vi "XY_plot_BW_gnuplot_DFT.vi"(0 "Plot Array":cluster{dbl[], dbl[]}[](array[cluster])=[{[-60.0, -57.5, -55.0, -52.5, -50.0, -47.5, -45.0, -42.5, -40.0, -37.5, -35.0, -32.5, -30.0, -27.5, -25.0, -22.5, -20.0, -17.5, -15.0, -12.5, -10.0, -7.5, -5.0, -2.5, 0.0, 2.5, 5.0, 7.5, 10.0, 12.5, 15.0, 17.5, 20.0, 22.5, 25.0, 27.5, 30.0, 32.5, 35.0, 37.5, 40.0, 42.5, 45.0, 47.5, 50.0, 52.5, 55.0, 57.5, 60.0], [0.6926572, 0.7210577, 0.7336973, 0.7296005, 0.7065726, 0.6675372, 0.6509055, 0.666809, 0.7019418, 0.7280011, 0.7366155, 0.7266001, 0.6985851, 0.6651901, 0.6448196, 0.6503613, 0.6875361, 0.7183487, 0.7265879, 0.7127957, 0.6835807, 0.6433804, 0.621768, 0.6334316, 0.670315, 0.7004812, 0.7073965, 0.6966882, 0.6633028, 0.6324072, 0.6188318, 0.6325043, 0.6686596, 0.7028522, 0.7124769, 0.7009745, 0.6723148, 0.6300974, 0.6088247, 0.6211135, 0.6589306, 0.6947777, 0.7073037, 0.6986245, 0.6763866, 0.6414574, 0.6211717, 0.6351113, 0.6695351]}, {[-250.0, -245.0, -240.0, -235.0, -230.0, -225.0, -220.0, -215.0, -210.0, -205.0, -200.0, -195.0, -190.0, -185.0, -180.0, -175.0, -170.0, -165.0, -160.0, -155.0, -150.0, -145.0, -140.0, -135.0, -130.0, -125.0, -120.0, -115.0, -110.0, -105.0, -100.0, -95.0, -90.0, -85.0, -80.0, -75.0, -70.0, -65.0, -60.0, -55.0, -50.01, -45.0, -40.0, -35.0, -30.0, -25.0, -20.0, -15.0, -10.0, -5.0, 0.0, 5.0, 10.0, 15.0, 20.0, 25.0, 30.0, 35.0, 40.0, 45.0, 50.0, 55.0, 60.0, 65.0, 70.0, 75.0, 80.0, 85.0, 90.0, 95.0, 100.0, 105.0, 110.0, 115.0, 120.0, 125.0, 130.0, 135.0, 140.0, 145.0, 150.0, 155.0, 160.0, 165.0, 170.0, 175.0, 180.0, 185.0, 190.0, 195.0, 200.0, 205.0, 210.0, 215.0, 220.0, 225.0, 230.0, 235.0, 240.0, 245.0, 250.0], [0.6258228, 0.6506318, 0.6351729, 0.7010563, 0.666653, 0.6318866, 0.6418648, 0.6775528, 0.6772554, 0.6566841, 0.6714944, 0.6985058, 0.678455, 0.6443694, 0.6531426, 0.6719725, 0.6524493, 0.6260805, 0.64483, 0.6829994, 0.659875, 0.6199248, 0.6366962, 0.6786398, 0.6778554, 0.6498207, 0.6635327, 0.6868778, 0.6697222, 0.641235, 0.6519968, 0.6776285, 0.6615762, 0.6471135, 0.6708456, 0.6800422, 0.6428301, 0.6228845, 0.6529464, 0.6825998, 0.6581101, 0.6411269, 0.673482, 0.6917087, 0.6575879, 0.6369717, 0.6618911, 0.6765118, 0.6419686, 0.6179553, 0.6401561, 0.6835365, 0.6558098, 0.6374033, 0.6669807, 0.6870508, 0.6587676, 0.6427578, 0.6715876, 0.6928693, 0.6606558, 0.6407446, 0.6661822, 0.6808485, 0.649376, 0.6387559, 0.6726195, 0.6840063, 0.6428675, 0.6274834, 0.6671746, 0.6892811, 0.6632424, 0.6494314, 0.6844879, 0.7061464, 0.667844, 0.6523467, 0.6754834, 0.6831993, 0.6537409, 0.650146, 0.6863526, 0.6915197, 0.6527784, 0.6421613, 0.6812965, 0.7003779, 0.6678409, 0.6625075, 0.6991244, 0.6979552, 0.658929, 0.6426513, 0.6723225, 0.6756767, 0.6454689, 0.6509592, 0.6810775, 0.6720489, 0.6356013]}, {[-250.0, -245.0, -240.0, -235.0, -230.0, -225.0, -220.0, -215.0, -210.0, -205.0, -200.0, -195.0, -190.0, -185.0, -180.0, -175.0, -170.0, -165.0, -160.0, -155.0, -150.0, -145.0, -140.0, -135.0, -130.0, -125.0, -120.0, -115.0, -110.0, -105.0, -100.0, -95.0, -90.0, -85.0, -80.0, -75.0, -70.0, -65.0, -60.0, -55.0, -50.0, -45.0, -40.0, -35.0, -30.0, -25.0, -20.0, -15.0, -10.0, -5.0, 0.0, 5.0, 10.0, 15.0, 20.0, 25.0, 30.0, 35.0, 40.0, 45.0, 50.0, 55.0, 60.0, 65.0, 70.0, 75.0, 80.0, 85.0, 90.0, 95.0, 100.0, 105.0, 110.0, 115.0, 120.0, 125.0, 130.0, 135.0, 140.0, 145.0, 150.0, 155.0, 160.0, 165.0, 170.0, 175.0, 180.0, 185.0, 190.0, 195.0, 200.0, 205.0, 210.0, 215.0, 220.0, 225.0, 230.0, 235.0, 240.0, 245.0, 250.0], [0.7199633, 0.71586, 0.7146621, 0.720776, 0.7208473, 0.7155022, 0.7097559, 0.7138091, 0.7261716, 0.7358918, 0.7412903, 0.7471439, 0.7430872, 0.7318501, 0.7242517, 0.7215749, 0.7168437, 0.7096065, 0.7113085, 0.7181352, 0.7186632, 0.7101602, 0.7056491, 0.713961, 0.727691, 0.7317399, 0.7345805, 0.7315234, 0.7289434, 0.7173446, 0.7110098, 0.7114931, 0.7136913, 0.7211985, 0.72029, 0.7193148, 0.7070549, 0.6992863, 0.7012733, 0.7126021, 0.7232668, 0.7273864, 0.7349982, 0.7363434, 0.7267652, 0.7217994, 0.7205206, 0.7193069, 0.7106847, 0.6995876, 0.6970152, 0.7001581, 0.6993276, 0.6998134, 0.7069099, 0.7110891, 0.7119888, 0.7107461, 0.7153481, 0.7219045, 0.714913, 0.7080906, 0.7068127, 0.7038392, 0.698503, 0.7005704, 0.7003845, 0.7038539, 0.6953904, 0.6920397, 0.7001599, 0.7094703, 0.7137769, 0.7180073, 0.7230059, 0.7250995, 0.7213451, 0.7111041, 0.7094518, 0.7083167, 0.7040226, 0.7066045, 0.7097009, 0.7077949, 0.7014225, 0.7058737, 0.7102084, 0.7183272, 0.7217187, 0.7251733, 0.7275464, 0.7183908, 0.7059657, 0.7016548, 0.7006334, 0.702877, 0.7023345, 0.7034203, 0.7042745, 0.698976, 0.6924951]}, {[-250.0, -245.0, -240.0, -235.0, -230.0, -225.0, -220.0, -215.0, -210.0, -205.0, -200.0, -195.0, -190.0, -185.0, -180.0, -175.0, -170.0, -165.0, -160.0, -155.0, -150.0, -145.0, -140.0, -135.0, -130.0, -125.0, -120.0, -115.0, -110.0, -105.0, -100.0, -95.0, -90.0, -85.0, -80.0, -75.0, -70.0, -65.0, -60.0, -55.0, -50.0, -45.0, -40.0, -35.0, -30.0, -25.0, -20.0, -15.0, -10.0, -5.0, 0.0, 5.0, 10.0, 15.0, 20.0, 25.0, 30.0, 35.0, 40.0, 45.0, 50.0, 55.0, 60.0, 65.0, 70.0, 75.0, 80.0, 85.0, 90.0, 95.0, 100.0, 105.0, 110.0, 115.0, 120.0, 125.0, 130.0, 135.0, 140.0, 145.0, 150.0, 155.0, 160.0, 165.0, 170.0, 175.0, 180.0, 185.0, 190.0, 195.0, 200.0, 205.0, 210.0, 215.0, 220.0, 225.0, 230.0, 235.0, 240.0, 245.0, 250.0], [0.768425, 0.7646976, 0.7648598, 0.7620641, 0.7619677, 0.7591337, 0.7573157, 0.7577341, 0.7682732, 0.7776914, 0.7864129, 0.7911217, 0.7902806, 0.7870794, 0.7748631, 0.7664278, 0.7640868, 0.7634201, 0.7630689, 0.7622264, 0.7616281, 0.763408, 0.764395, 0.7665321, 0.771622, 0.7807466, 0.7826597, 0.784532, 0.7764856, 0.7691938, 0.7589803, 0.7538694, 0.7541752, 0.7570843, 0.7569958, 0.753328, 0.7533831, 0.7480442, 0.7493855, 0.7557662, 0.768794, 0.7812232, 0.7894507, 0.7928332, 0.7911097, 0.7813342, 0.7759887, 0.7691784, 0.7640505, 0.7602281, 0.7583228, 0.753628, 0.7548767, 0.7528715, 0.7584033, 0.7654095, 0.7705307, 0.7787003, 0.7801007, 0.7821146, 0.7765937, 0.768884, 0.7656759, 0.7562703, 0.7536232, 0.7539161, 0.7465613, 0.7489434, 0.7465653, 0.7487705, 0.7513418, 0.7602761, 0.771601, 0.779764, 0.7822907, 0.78155, 0.7763815, 0.7693112, 0.7626131, 0.7605712, 0.7588274, 0.7591805, 0.7584174, 0.7597108, 0.7548346, 0.7577244, 0.7606031, 0.7694007, 0.7775843, 0.7796888, 0.7780972, 0.7765036, 0.7638986, 0.760308, 0.7578089, 0.7541802, 0.7539944, 0.7565544, 0.7576207, 0.7557231, 0.7539951]}, {[-250.0, -240.0, -230.0, -220.0, -210.0, -200.0, -190.0, -180.0, -170.0, -160.0, -150.0, -140.0, -130.0, -120.0, -110.0, -100.0, -90.0, -80.0, -70.0, -60.0, -50.0, -40.0, -30.0, -20.0, -10.0, 0.0, 10.0, 20.0, 30.0, 40.0, 50.0, 60.0, 70.0, 80.0, 90.0, 100.0, 110.0, 120.0, 130.0, 140.0, 150.0, 160.0, 170.0, 180.0, 190.0, 200.0, 210.0, 220.0, 230.0, 240.0, 250.0], [0.7802652, 0.7730503, 0.7695233, 0.768015, 0.7807572, 0.7935942, 0.7974301, 0.7898797, 0.7780562, 0.7727421, 0.7754456, 0.7827163, 0.792625, 0.796434, 0.7864364, 0.7709765, 0.7651486, 0.7583434, 0.7591986, 0.7686091, 0.7853258, 0.8037569, 0.8016167, 0.7895253, 0.7775238, 0.7695855, 0.7682042, 0.7766473, 0.7899663, 0.7972402, 0.7915579, 0.78097, 0.7681623, 0.7627507, 0.7612609, 0.7754872, 0.7942263, 0.8006955, 0.7949862, 0.7807588, 0.7743586, 0.7702566, 0.7745907, 0.7822656, 0.7926563, 0.7935593, 0.7845497, 0.7732503, 0.7678837, 0.7717659, 0.773242]}, {[-250.0, -240.0, -230.0, -220.0, -210.0, -200.0, -190.0, -180.0, -170.0, -160.0, -150.0, -140.0, -130.0, -120.0, -110.0, -100.0, -90.0, -80.0, -70.0, -60.0, -50.0, -40.0, -30.0, -20.0, -10.0, 0.0, 10.0, 20.0, 30.0, 40.0, 50.0, 60.0, 70.0, 80.0, 90.0, 100.0, 110.0, 120.0, 130.0, 140.0, 150.0, 160.0, 170.0, 180.0, 190.0, 200.0, 210.0, 220.0, 230.0, 240.0, 250.0], [0.7879372, 0.7788166, 0.7776735, 0.7776241, 0.7889971, 0.8028856, 0.8070604, 0.8038303, 0.7927997, 0.7844949, 0.7865187, 0.7911869, 0.8018413, 0.8059924, 0.7943886, 0.7807321, 0.7705954, 0.7683053, 0.7699354, 0.779466, 0.7983266, 0.8136788, 0.8131328, 0.8038514, 0.7875963, 0.7800124, 0.7816548, 0.7885765, 0.8014482, 0.8085178, 0.8013688, 0.7883396, 0.7755844, 0.7736845, 0.7744691, 0.7907869, 0.8086567, 0.8114194, 0.8067535, 0.7936511, 0.7873925, 0.7810313, 0.7904059, 0.7965633, 0.8057665, 0.8044745, 0.7962059, 0.788702, 0.7812019, 0.7861557, 0.7902221]}, {[-250.0, -240.0, -230.0, -220.0, -210.0, -200.0, -190.0, -180.0, -170.0, -160.0, -150.0, -140.0, -130.0, -120.0, -110.0, -100.0, -90.0, -80.0, -70.0, -60.0, -50.0, -40.0, -30.0, -20.0, -10.0, 0.0, 10.0, 20.0, 30.0, 40.0, 50.0, 60.0, 70.0, 80.0, 90.0, 100.0, 110.0, 120.0, 130.0, 140.0, 150.0, 160.0, 170.0, 180.0, 190.0, 200.0, 210.0, 220.0, 230.0, 240.0, 250.0], [0.8154395, 0.8122923, 0.8086691, 0.8108997, 0.8191707, 0.8265118, 0.8294095, 0.8293452, 0.822631, 0.8238484, 0.8233996, 0.8241853, 0.8276184, 0.8234715, 0.8165378, 0.8082245, 0.798939, 0.798317, 0.8042167, 0.8193354, 0.8322321, 0.8402989, 0.8372588, 0.8290143, 0.8194996, 0.8153282, 0.8137867, 0.821221, 0.8254559, 0.8235515, 0.8236829, 0.8128044, 0.8098797, 0.8100971, 0.8177005, 0.8258541, 0.8346069, 0.8371071, 0.8288949, 0.8221575, 0.8182937, 0.8175638, 0.8224113, 0.8234351, 0.8289554, 0.824578, 0.819657, 0.8128183, 0.8152596, 0.8195102, 0.8255393]}, {[-250.0, -240.0, -230.0, -220.0, -210.0, -200.0, -190.0, -180.0, -170.0, -160.0, -150.0, -140.0, -130.0, -120.0, -110.0, -100.0, -90.0, -80.0, -70.0, -60.0, -50.0, -40.0, -30.0, -20.0, -10.0, 0.0, 10.0, 20.0, 30.0, 40.0, 50.0, 60.0, 70.0, 80.0, 90.0, 100.0, 110.0, 120.0, 130.0, 140.0, 150.0, 160.0, 170.0, 180.0, 190.0, 200.0, 210.0, 220.0, 230.0, 240.0, 250.0], [0.83059, 0.8293368, 0.8266022, 0.8290301, 0.8318731, 0.8391975, 0.8396511, 0.8408702, 0.8420259, 0.8377043, 0.837982, 0.8357183, 0.8335366, 0.8289886, 0.8236064, 0.8201522, 0.8188415, 0.8206514, 0.8238208, 0.8296316, 0.8366576, 0.8424445, 0.8437929, 0.8414023, 0.8376481, 0.8330458, 0.8310008, 0.8321893, 0.8334765, 0.832358, 0.8307255, 0.8322423, 0.8301097, 0.8318011, 0.8373023, 0.8428455, 0.8447038, 0.843124, 0.8437177, 0.8434732, 0.8408547, 0.8400876, 0.8407896, 0.8403817, 0.8420662, 0.8382707, 0.8379485, 0.8372055, 0.8393238, 0.8426629, 0.8465353]}] {"?" format="%.2f"; "?" format="%.2f"}, 1 "Job Directory":path=path "/G5_1_HD/Users/paulhayden/Desktop/Ryan/8-5-06") -> (2 "Saved Automatically?":bool, 3 "Tex Info String":string="set term epslatex\nset output \"Plot.eps\"\nset xlabel '$Wavelength~[mm]$'\nset ylabel '$U/Ur~Spectral~energy$'\nset samples 1000\nset pointsize 1.00\nset title '$$' 0, 0\nset size 0.75,2.5\n\n#set key 225, -696.080\n unset key\n set xrange [0 : 250] \n# set autoscale x \n set yrange [-602 : 84]\n# set autoscale y \nset ytics (\"x/h=313\" 0,\"x/h=218\" -84,\"x/h=124\" -168,\"x/h=102\" -252,\"x/h=66\" -336,\"x/h=34\" -420,\"x/h=18\" -504,\"x/h=10\" -588)\n\nplot \"Spec_U_Ur_x_h_10_x_h_18d.dat\" index 0 using 1:2 axes x1y1 title '$x/h=313$' with linespoints, \\\n\"Spec_U_Ur_x_h_10_x_h_18d.dat\" index 1 using 1:2 axes x1y1 title '$x/h=218$' with linespoints, \\\n\"Spec_U_Ur_x_h_10_x_h_18d.dat\" index 2 using 1:2 axes x1y1 title '$x/h=124$' with linespoints, \\\n\"Spec_U_Ur_x_h_10_x_h_18d.dat\" index 3 using 1:2 axes x1y1 title '$x/h=102$' with linespoints, \\\n\"Spec_U_Ur_x_h_10_x_h_18d.dat\" index 4 using 1:2 axes x1y1 title '$x/h=66$' with linespoints, \\\n\"Spec_U_Ur_x_h_10_x_h_18d.dat\" index 5 using 1:2 axes x1y1 title '$x/h=34$' with linespoints, \\\n\"Spec_U_Ur_x_h_10_x_h_18d.dat\" index 6 using 1:2 axes x1y1 title '$x/h=18$' with linespoints, \\\n\"Spec_U_Ur_x_h_10_x_h_18d.dat\" index 7 using 1:2 axes x1y1 title '$x/h=10$' with linespoints", 4 "Plot data file":path)   [LabVIEW 2010]
uses:
  Results_plotter_Global.vi
  <vilib>/Analysis/NI_AALBase.lvlib
  <vilib>/Analysis/NI_AALPro.lvlib
  Gnuplot_Label.ctl
  Analysis/Windowing_list.ctl
  Analysis/Mean_shift_list.ctl
  Analysis/Autocorrelation_list.ctl
panel:
  in  "Case Constant\n(See Context Help) 2":bool
  in  "Case Constant\n(See Context Help)":bool
  in  "Autocorrelation before DFT":T1=enum."Biased"
  in  "Fmin Factor":dbl(knob)=1.5 scale=1.0..9.0
  in  "Mean shifting":T2=enum."Eliminate DC only"
  in  "Freq?":bool
  in  "DF Factor":i32(knob)=5 scale=1.0..9.0
  in  "Window Type":T3
  in  "fmax":dbl=30.0
  out "Final Title":string
  in  "Tweak scale":bool
  in  "y Log?":bool
  in  "Show keep Dialog?":bool
  in  "Mode":T4=enum."Only Bottom Label"
  in  "Wavelenght?":bool
  in  "Separation":dbl=1.2
  in  "Reverse order":bool=TRUE
  in  "Offset?":bool=TRUE
  out "Extra range":dbl=602.0
  in  "precision":string
  out "Profile offset":dbl=70.0
  in  "Graph Height":string="2.5"
  in  "Graph width":string="0.75"
  in  "Filename Max length":i32=28
  in  "Save data analysis file":bool=TRUE
  in  "Plot Title":u16(ring) items=["Title String Only", "File::", "::x [mm]", "::y [mm]", "::z [mm]", "::z/delta", "x/h::", "::Uo", "::Ur", "::Ur/Uo", "::U/Uo", "XW:Calibration:Drift", "Date:of:Measurement", "Measurement:Type:", "Average:Sampling:Rate [Hz]", "Original:Results:Filename", "Comments::", "Leading Edge::", "Roughness:Pattern:", "Roughness:Element:", "Roughness:Element:Height (mm)", "Roughness:Area:Density (%)", "Roughness:Baseboard:Floor Ht [mm]", "X Offset::", "Reference:Temperature:Deg C", "::Uo/Ulocal", "BL:Depth:[mm]", "U/Ur:Profile:Sigma"]
  in  "Plot style":u16[](array[ring])=[2, 2, 2, 2, 2, 2, 2, 2, 2] items=["points", "lines", "linespoints"]
  in  "Summarise":u16(ring) items=["All Series", "x/h=152; ", "x/h=132; ", "x/h=112; ", "x/h=92; ", "x/h=80; ", "x/h=52; ", "x/h=35; ", "x/h=18; ", "x/h=11; "]
  in  "Added labels":i32[](listbox)
  out "Delta y":dbl=67.2
  out "Y location":dbl=-696.0799999999999
  out "X location":dbl=-50.0
  in  "Plot Title":string
  in  "Show legend?":bool
  in  "Point Size":dbl=1.0 format="%.2f"
  out "No of Series":i32=8
  in  "Fit type":T5(ring)
  out "No Legend":i32=397
  out "With legend":i32=580
  in  "Auto scale?":bool
  out "Current filename index":i32=-1
  in  "Save Automatically?":bool=TRUE
  in  "Analysis":T6(ring)=enum."Spectrum"
  out "XY Graph":cluster{dbl[], dbl[]}[](graph)=[{[333.3333333333333, 294.7976878612717, 264.24870466321244, 239.43661971830988, 218.8841201716738, 201.5810276679842, 186.81318681318683, 174.06143344709895, 162.93929712460064, 153.15315315315314, 144.47592067988668, 136.72922252010724, 129.77099236641223, 123.48668280871672, 117.78290993071593, 112.58278145695365, 107.82241014799155, 103.44827586206895, 99.41520467836258, 95.68480300187618, 92.2242314647378, 89.00523560209425, 86.00337268128162, 83.1973898858075, 80.56872037914692, 78.1010719754977, 75.78008915304606, 73.5930735930736, 71.52875175315567, 69.57708049113234, 67.72908366533865, 65.97671410090557, 64.31273644388398, 62.73062730627306, 61.22448979591837, 59.78898007033998, 58.419243986254294, 57.110862262038076, 55.85980284775465, 54.66237942122187, 53.51521511017839, 52.41521068859198, 51.35951661631421, 50.34550839091807, 49.370764762826724, 48.433048433048434, 47.53028890959926, 46.660567246111626, 45.82210242587602, 45.013239187996476, 44.232437120555076, 43.47826086956522, 42.74937133277452, 42.04451772464963, 41.36253041362531, 40.702314445331204, 40.062843676355065, 39.4431554524362, 38.84234577303884, 38.25956489122281, 37.6940133037694, 37.144938091769845, 36.6116295764537, 36.09341825902336, 35.58967201674808, 35.09979353062629, 34.623217922606926, 34.15941058271936, 33.70786516853933, 33.268101761252446, 32.83966516419833, 32.42212333121424, 32.015065913371004, 31.61810291382517, 31.23086344151868, 30.8529945553539, 30.484160191273162, 30.12404016538689, 29.7723292469352, 29.428736295441432, 29.092983456930973, 28.764805414551606, 28.443948689347458, 28.130170987313843, 27.823240589198036, 27.52293577981651, 27.229044313934864, 26.941362916006337, 26.659696811291166, 26.38385928608381, 26.113671274961597, 25.848960973137356, 25.58956347215253, 25.33532041728763, 25.086079685194296, 24.84169508037019, 24.602026049204053, 24.36693741041567, 24.136299100804543, 23.90998593530239, 23.687877380399442, 23.469857340082836, 23.25581395348837, 23.04563940352463, 22.839229735781462, 22.636484687083886, 22.43730752309723, 22.241604884430874, 22.04928664072633, 21.86026575225032, 21.674458138546534, 21.491782553729458, 21.312160468031756, 21.135515955242436, 20.96177558569667, 20.79086832450061, 20.622725434694704, 20.457280385078217, 20.294468762435336, 20.134228187919465, 19.976498237367803], [0.5990496790577843, 0.10204934004139832, 0.0019233437344699468, 0.0015283816083073542, 0.1404030678688706, 0.932862399424205, 2.8050868438053804, 6.206466594164352, 12.174974271095522, 20.7873605572333, 27.752136534354648, 26.187079474414283, 16.066183198458866, 5.855400131907148, 1.1502873482765865, 0.14978933164687652, 0.06507388251633289, 0.08545959621434393, 0.0606820076976982, 0.020062596633821553, 0.01049802299219501, 0.021411252916291184, 0.03838230643884463, 0.05403742233599998, 0.11728907089858254, 0.33817560027039006, 0.7088104156694127, 0.8444536593716904, 0.518995682293636, 0.14222804476121165, 0.014816837096635968, 0.004801288194402382, 0.018694308160986207, 0.028238928408325002, 0.011132390574814957, 0.00047033266820432706, 5.12975108150408e-05, 0.0041267067349246705, 0.014442143511050337, 0.014240376853560659, 0.005759524814622401, 0.001546648037191398, 0.0010963414467816998, 0.001723590800103069, 0.00198485071072457, 0.0020070371956419667, 0.0030201156383263417, 0.005238532043374439, 0.006190957277067641, 0.003934285647612388, 0.001183674416189446, 0.00016024743898354163, 2.9538490837431888e-05, 3.5022386095358224e-05, 2.5068161892268835e-05, 2.5056543858637915e-06, 2.965222646731639e-07, 3.646397650845149e-05, 0.00036526317218077897, 0.00146249813968966, 0.003359341451077737, 0.0047098164852658955, 0.003971612726124136, 0.0020223318392337607, 0.000777352151228649, 0.00045658307393260785, 0.0004509571774923791, 0.00027299932161513004, 3.276133714704423e-05, 3.561764806155004e-07, 0.00011669097888005772, 0.0008205935740738643, 0.0012506042598999568, 0.0005459090002590769, 4.588878406552742e-05, 3.0600893268824806e-05, 0.0004580825578230784, 0.0012572934478299537, 0.0009403278349473496, 0.0001513751720034608, 2.8773674135653848e-06, 0.00012788979408662275, 0.0009628787005658209, 0.0016491692919722988, 0.001025218593828607, 0.000259108954298406, 7.555698716651012e-05, 0.00020924662382651018, 0.000635441834449123, 0.0009234992226142822, 0.000685824239809675, 0.000252171148113808, 3.0441503964447473e-05, 5.5007155443445065e-08, 2.5448796911200823e-06, 3.5604093485379316e-05, 4.953185709102323e-05, 8.464211723874017e-06, 4.863386637333031e-08, 5.814431200530514e-05, 0.0005637692199884538, 0.0012280895581986383, 0.0008855968153969191, 0.00016783367601854734, 7.995389181969868e-06, 9.744157884719188e-05, 0.0005605518200691667, 0.0006393664152836468, 0.00013128671333363014, 6.009241375369227e-08, 8.31083729047157e-05, 0.0010228372037594281, 0.00200215465382885, 0.0011548837367990228, 0.00018046416728848235, 5.202104238264702e-05, 0.0004147741794859646, 0.001131022279409099, 0.0008255052061356253, 0.00013780101939323442, 2.2264774482623323e-05]}, ...(8 in all)]
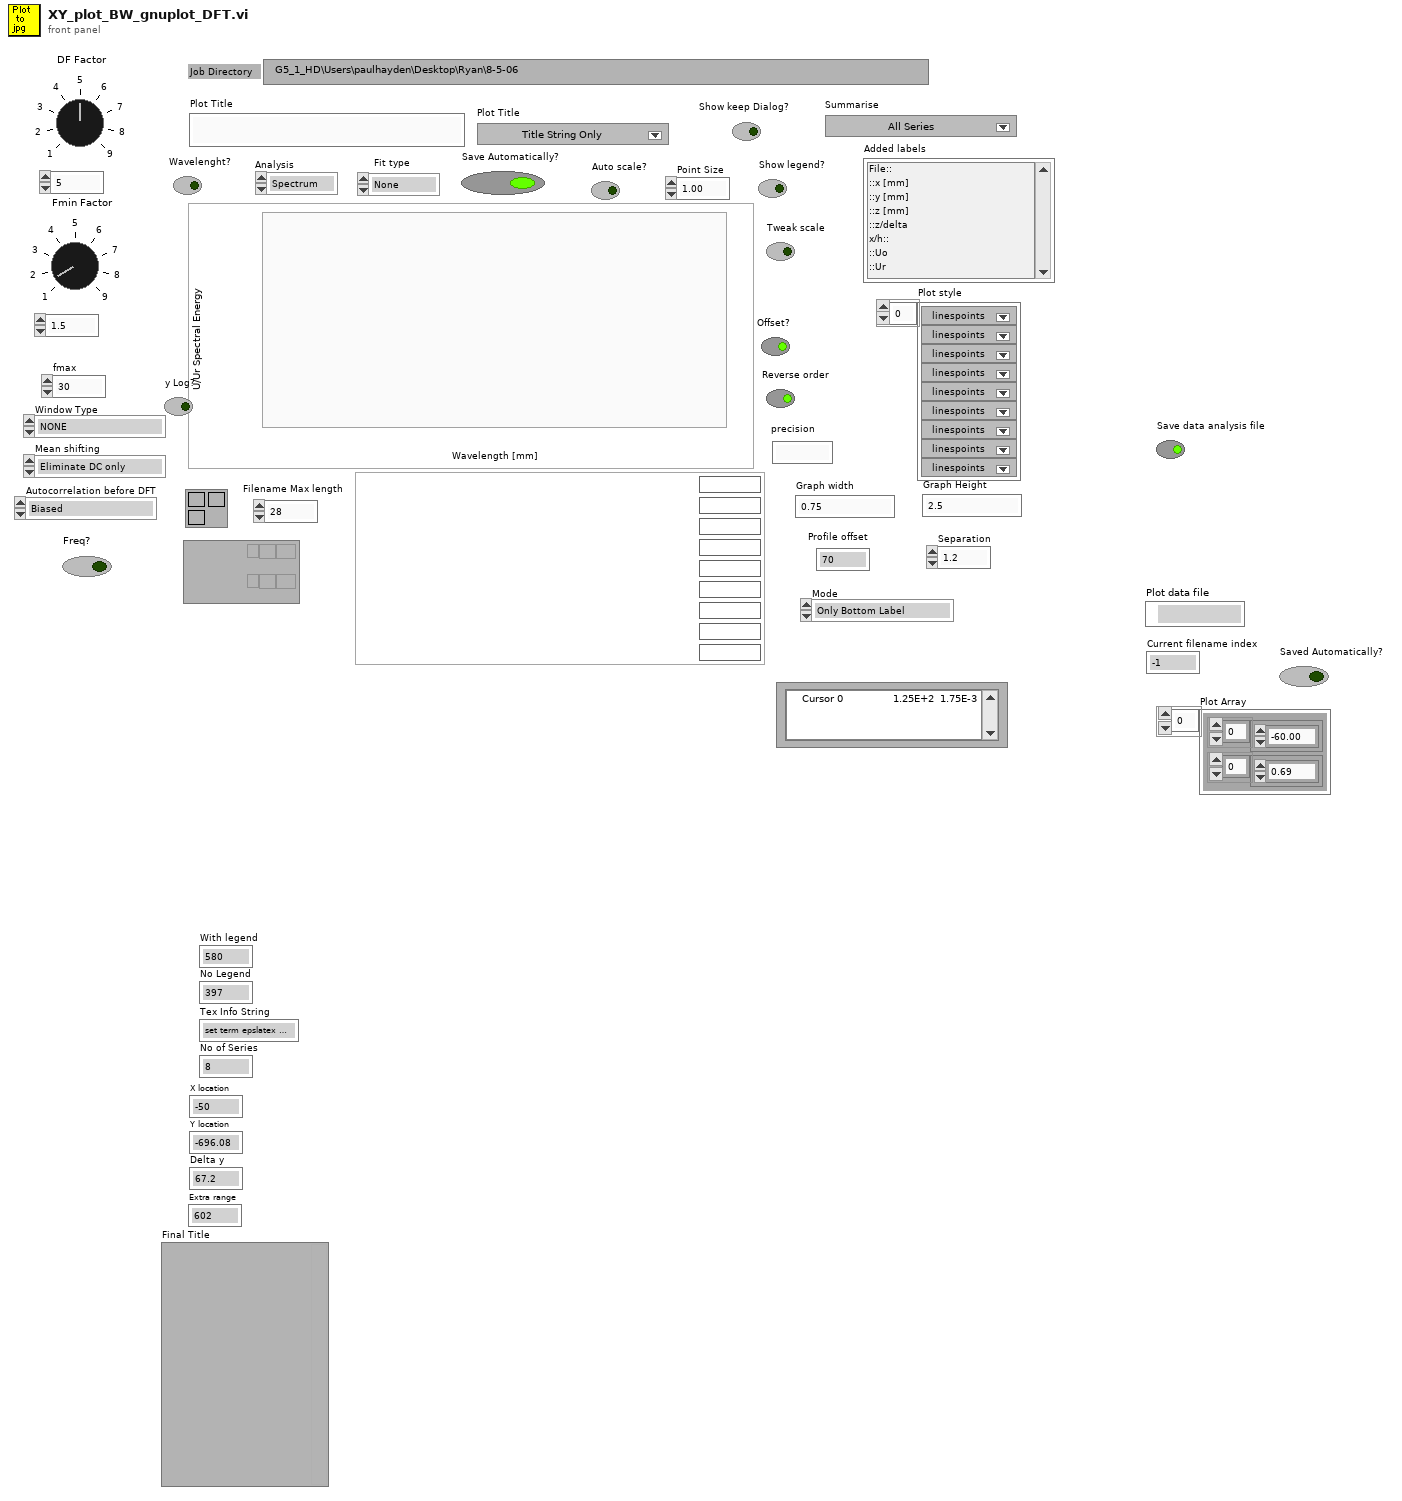
[diagram p1: front panel]
types:
  T1 = typedef "Autocorrelation_list.ctl" = enum16{"NONE", "Biased", "Un-biased"}
  T2 = typedef "Mean_shift_list.ctl" = enum16{"NONE", "Eliminate DC only", "Eliminate all linear trends"}
  T3 = typedef "Windowing_list.ctl" = enum16{"NONE", "Blackman", "Blackman Harris", "Cosine Taper", "Exact Blackman", "Flat Top", "Hamming", "Hanning", "Sine", "Triangle"}
  T4 = typedef "Gnuplot_Label.ctl" = enum16{"3 Labels per plot", "Only Center label", "Only Bottom Label"}
  T5 = enum16{"None", "Lines", "Linespoints", "Spline", "Linear", "2nd Ploy", "3rd Poly", "4th Poly", "Gaussian"}
  T6 = enum16{"None", "% change", "Spectrum", "Norm Spec"}
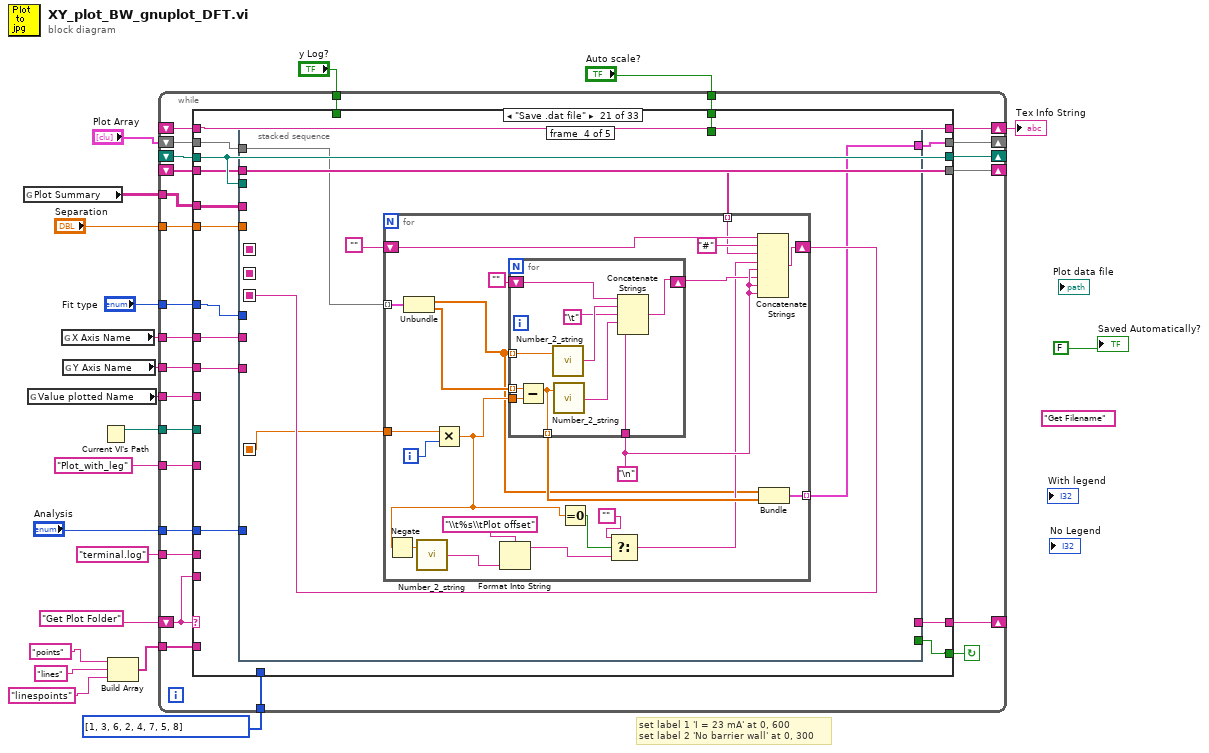
[diagram p0: block diagram]
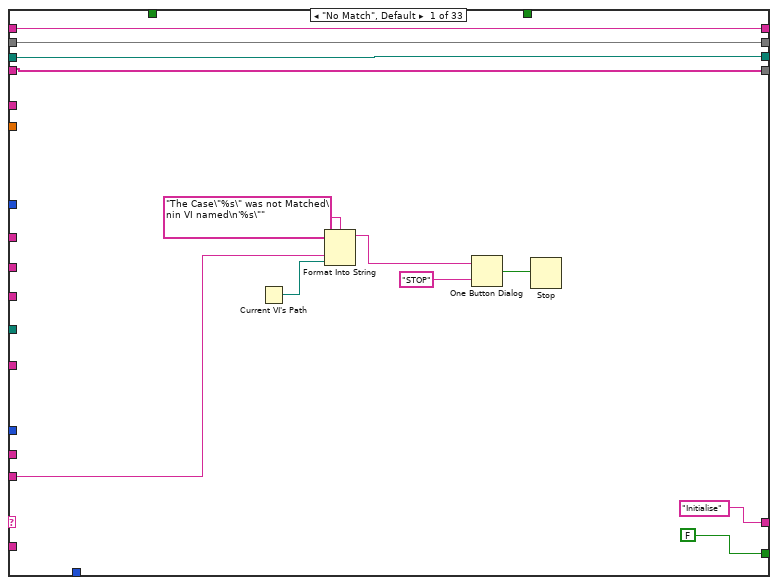
[diagram p2: hidden frame]
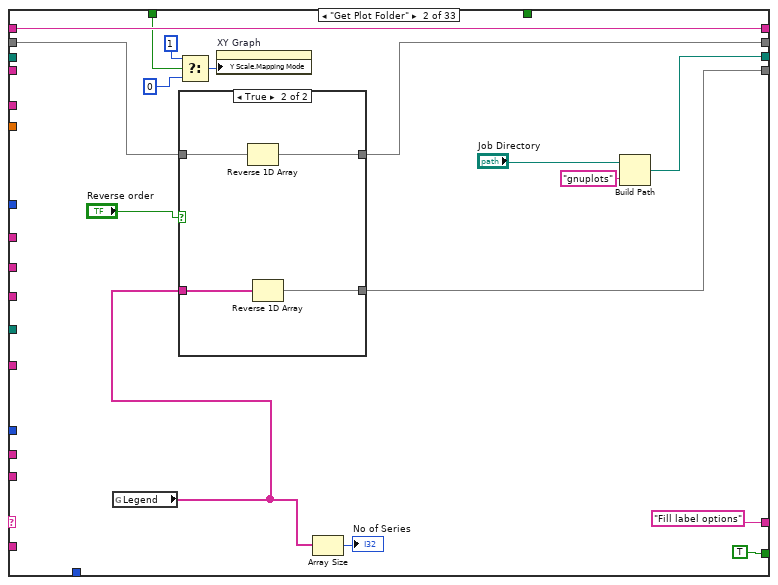
[diagram p3: hidden frame]
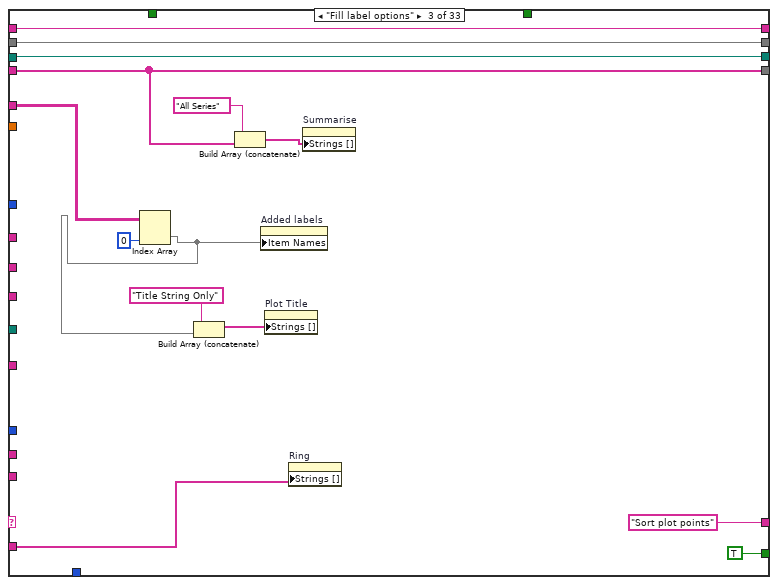
[diagram p5: hidden frame]
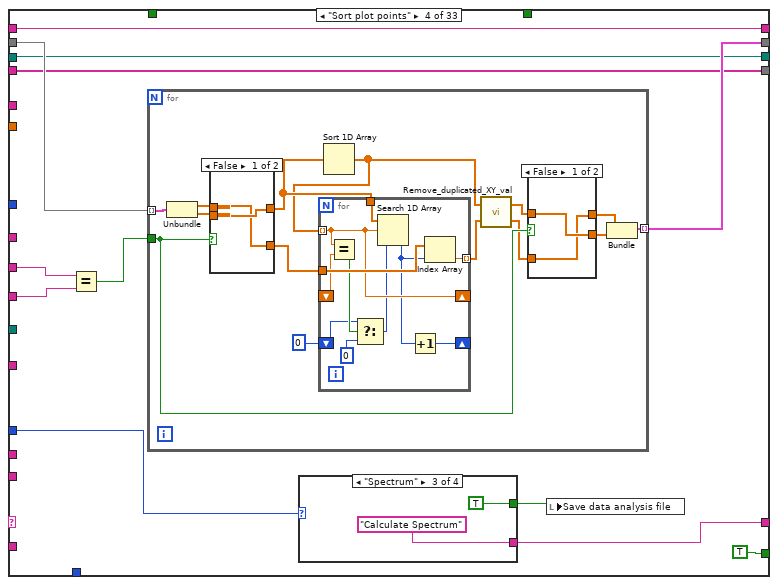
[diagram p6: hidden frame]
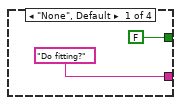
[diagram p7: hidden frame]
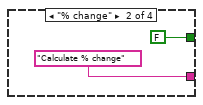
[diagram p8: hidden frame]
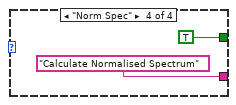
[diagram p9: hidden frame]
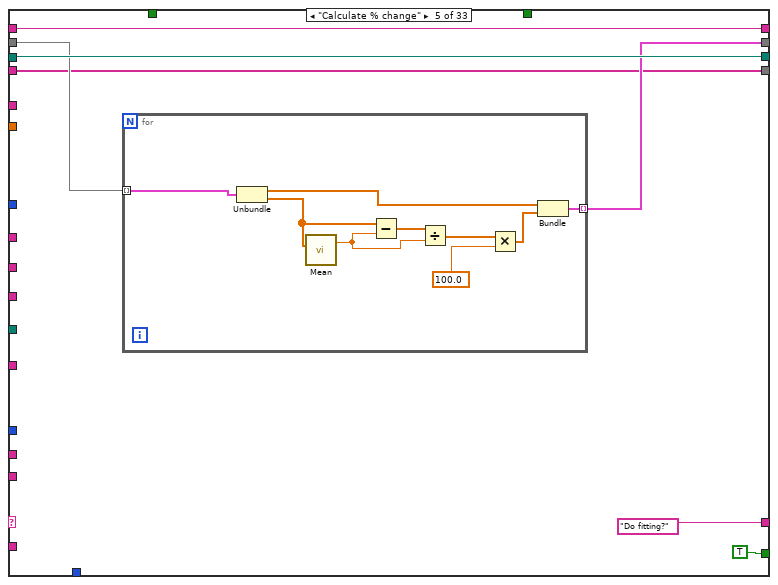
[diagram p12: hidden frame]
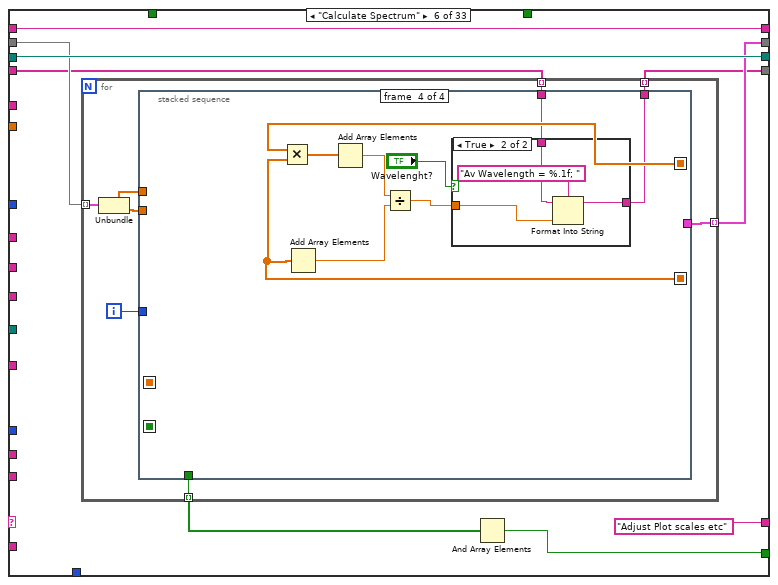
[diagram p13: hidden frame]
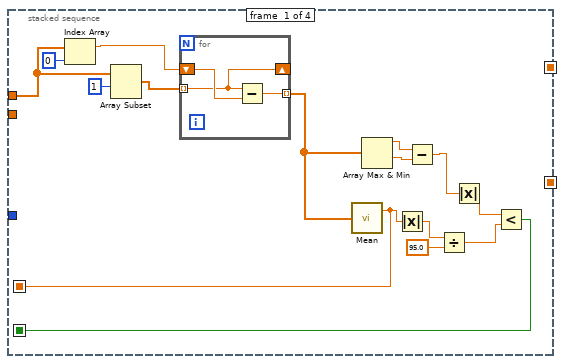
[diagram p14: hidden frame]
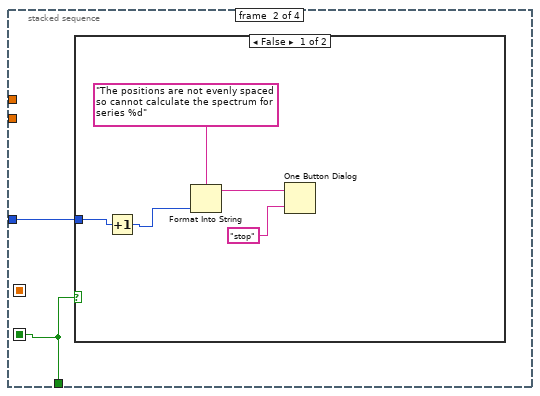
[diagram p15: hidden frame]
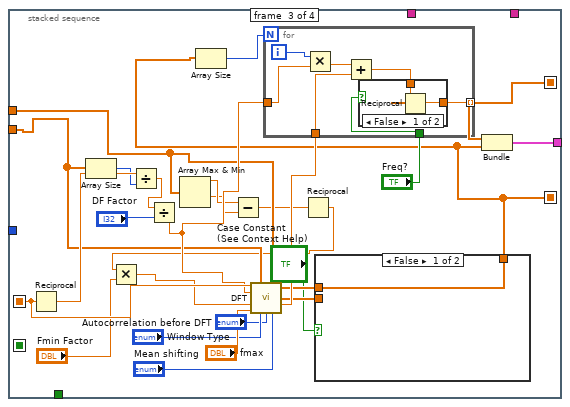
[diagram p17: hidden frame]
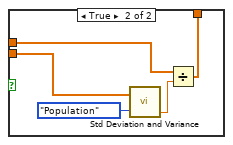
[diagram p18: hidden frame]
diagram:
  (unwired) "Get Filename"
  # "set label 1 'I = 23 mA' at 0, 600\nset label 2 'No barrier wall' at 0, 300"
  n1 = global read "Results_plotter_Global.vi" "Plot Summary"() -> (w19:string[][])
  n2 = global read "Results_plotter_Global.vi" "Value plotted Name"() -> (w16:string)
  n3 = global read "Results_plotter_Global.vi" "X Axis Name"() -> (w18:string)
  n4 = global read "Results_plotter_Global.vi" "Y Axis Name"() -> (w17:string)
  n5 = Current VI's Path() -> (path=w20:path)
  n6 = Build Array("points", "lines", "linespoints") -> (w5:string[])
  n7 = while {
    shift-left: "Get Plot Folder" -> [w44]
    shift-right: [w45] -> _
    tunnel: w20 -> [w43]
    tunnel: w19 -> [w42]
    shift-right: [w41] -> _
    shift-left: _ -> [w40]
    tunnel: "Analysis" -> [w39]
    tunnel: w18 -> [w38]
    tunnel: w17 -> [w37]
    tunnel: w16 -> [w36]
    tunnel: "Auto scale?" -> [w35]
    shift-right: [w33] -> _
    shift-left: "Plot Array" -> [w34]
    shift-right: [w31] -> w13
    shift-left: _ -> [w32]
    tunnel: "Plot_with_leg" ("name or relative path") -> [w30]
    tunnel: "Fit type" -> [w29]
    shift-right: [w28] -> _
    shift-left: _ -> [w27]
    tunnel: "terminal.log" -> [w26]
    tunnel: w5 -> [w25]
    tunnel: i32[] [1, 3, 6, 2, 4, 7, 5, 8] ("Plot style") -> [w24]
    tunnel: "Separation" -> [w23]
    tunnel: "y Log?" -> [w22]
    stop <- w46 continue-if-true
    n8 = case shown="\"Save .dat file\"" w44 {
      tunnel: [FALSE TRUE TRUE ("Top Level") TRUE TRUE w166 w263 TRUE TRUE TRUE ("Top Level") TRUE ("Top Level") TRUE ("Top Level") TRUE ("Top Level") TRUE ("Top Level") w503 TRUE ("Top Level") TRUE ("Top Level") TRUE ("Top Level") TRUE ("Top Level") w719 w792 TRUE ("Top Level") TRUE ("Top Level") TRUE ("Top Level") TRUE ("Top Level") TRUE ("Top Level") TRUE ("Top Level") TRUE ("Top Level") TRUE ("Top Level") TRUE ("Top Level") "Show keep Dialog?" FALSE ("Top Level") FALSE ("Top Level")] -> w46
      tunnel: ["Initialise" "Fill label options" "Sort plot points" w96 "Do fitting?" "Adjust Plot scales etc" "Adjust Plot scales etc" "Adjust Plot scales etc" "Add fitted line styles" "Adjust Plot scales etc" w420 "Fill Second legend" "Fill Second legend" "Fill Second legend" w504 "Get Filename" ("t") w658 "Create plot directory" w701 w718 w791 "Edit Legend names" ("t") "Input Legend info" ("t") w969 w1076 w1179 "Plot Command" "Write gnuplot file" ("t") "Execute shell script" ("t") "Has pdf been generated?" ("t") w1366 "End" ("t") "End" ("t")] -> w45
      tunnel: w44 -> [w53 _ _ _ _ _ _ _ _ _ _ _ _ _ _ _ _ _ _ _ _ _ _ _ _ _ _ _ _ _ _ _ _]
      tunnel: w43 -> [_ _ _ _ _ _ _ _ _ _ _ _ _ _ w501 _ _ _ _ _ _ _ _ _ _ _ _ _ _ _ _ _ _]
      tunnel: w42 -> [_ _ w94 _ _ _ _ _ _ _ _ _ _ _ w502 w611 _ _ _ w717 w790 _ _ _ w1075 _ _ _ _ _ _ _ _]
      tunnel: [w50 w71 w88 w102 w152 w171 w269 w330 w345 w406 w433 w467 w476 w488 w500 w615 w659 w670 w703 w720 w793 w913 w944 w996 w1082 w1187 w1202 w1262 w1335 w1354 w1368 w1387 w1405] -> w41
      tunnel: w40 -> [w50 _ w88 w102 w152 w171 w269 w330 w345 w406 w433 w467 w476 w488 w496 w615 w655 w677 w704 w720 w793 w913 w944 w996 w1082 w1187 w1202 w1262 w1335 w1354 w1368 w1387 w1405]
      tunnel: w39 -> [_ _ _ w97 _ _ _ _ _ _ w421 _ _ w482 _ _ w646 _ _ w711 w783 w909 _ _ _ _ _ _ _ _ _ _ _]
      tunnel: w38 -> [_ _ _ _ _ _ _ _ w336 _ _ w466 w475 _ _ _ _ _ _ w716 w789 w907 _ _ _ _ _ _ _ _ _ _ _]
      tunnel: w37 -> [_ _ _ w100 _ _ _ _ w335 _ _ w462 w474 w487 _ _ _ _ _ w715 w788 w908 _ _ _ _ _ _ _ _ _ _ _]
      tunnel: w36 -> [_ _ _ w101 _ _ _ _ _ _ _ _ _ _ _ _ _ _ _ w710 _ _ _ _ _ _ _ _ _ _ _ _ _]
      tunnel: w35 -> [_ _ _ _ _ _ _ _ _ _ _ _ _ _ _ _ _ _ _ w713 w785 _ _ w980 _ w1182 _ _ _ _ _ _ _]
      tunnel: w34 -> [w49 w66 w89 w104 w151 w170 w268 w326 w341 w405 w419 w465 w473 w486 w499 w616 w657 w680 w707 w709 w787 w914 w938 w988 w1077 w1188 w1197 w1266 w1347 w1363 w1375 w1396 w1410]
      tunnel: [w49 w65 w89 w103 w150 w169 w267 w326 w334 w405 w419 w465 w473 w486 w499 w616 w657 w680 w707 w709 w782 w914 w938 w988 w1077 w1188 w1197 w1266 w1347 w1363 w1375 w1396 w1410] -> w33
      tunnel: w32 -> [w48 w70 w90 w99 w149 w168 w266 w329 w344 w403 w422 w464 w472 w485 w498 w607 w656 w679 w706 w721 w794 _ w943 w992 w1079 w1181 w1200 w1260 w1337 w1357 w1373 w1394 w1408]
      tunnel: [w48 w70 w90 w99 w149 w168 w266 w329 w344 w403 w422 w464 w472 w485 w498 w607 w656 w679 w706 w721 w794 w915 w943 w993 w1080 w1175 w1199 w1259 w1337 w1357 w1373 w1394 w1408] -> w31
      tunnel: w30 -> [_ _ _ _ _ _ _ _ _ _ _ _ _ _ _ _ _ _ _ _ _ _ _ _ _ _ _ _ _ _ _ _ _]
      tunnel: w29 -> [_ _ _ _ _ _ _ w327 w343 _ w424 _ _ _ _ _ _ _ _ w712 w784 _ _ _ _ w1180 w1204 w1251 _ _ _ _ _]
      tunnel: [w47 w63 w86 w98 w148 w164 w265 w328 w338 w402 w426 w463 w471 w484 w497 w614 w654 w678 w705 w714 w786 w912 w945 w995 w1081 w1168 w1205 w1261 w1336 w1362 w1374 w1395 w1409] -> w28
      tunnel: w27 -> [w47 _ w86 w98 w148 w165 w265 w328 w339 w402 w426 w463 w471 w484 w497 w614 w654 w678 w705 w714 w786 w912 w946 w995 w1081 w1168 w1205 w1261 w1336 w1362 w1374 w1395 w1409]
      tunnel: w26 -> [_ _ _ _ _ _ _ _ _ _ _ _ _ _ _ _ _ _ _ _ _ _ _ _ _ _ _ _ _ w1348 _ w1378 w1403]
      tunnel: w25 -> [_ _ w84 _ _ _ _ _ _ _ _ _ _ _ _ _ _ _ _ _ _ _ _ _ _ _ _ _ _ _ _ _ _]
      tunnel: w24 -> [_ _ _ _ _ _ _ _ _ _ _ _ _ _ _ _ _ _ _ _ _ _ _ _ _ _ _ w1249 w1332 _ _ _ _]
      tunnel: w23 -> [_ _ _ _ _ _ _ _ _ _ _ _ _ _ _ _ _ _ _ _ w781 _ w937 w960 _ w1165 _ _ _ _ _ _ _]
      tunnel: w22 -> [_ w62 _ _ _ _ _ _ _ _ _ _ _ _ _ _ _ _ _ _ _ _ _ w959 w1074 w1161 _ _ _ _ _ _ _]
      frame "No Match", Default {
        n9 = Current VI's Path() -> (path=w52:path)
        n10 = Format Into String(format string="The Case\"%s\" was not Matched\nin VI named\n'%s\"" ("Format String"), w53, w52) -> (resulting string=w56:string)  [unwired: 2 in, 1 out]
        n11 = One Button Dialog(message=w56, button name ("OK")="STOP") -> (true=w54:bool)
        n12 = Stop(stop? (T)=w54) -> ()
      }
      frame "Get Plot Folder" {
        n13 = global read "Results_plotter_Global.vi" "Legend"() -> (w64:string[])
        n14 = case shown="True" "Reverse order" {
          tunnel: w66 -> [w76 w80]
          tunnel: [w76 w79] -> w65
          tunnel: w64 -> [w75 w78]
          tunnel: [w75 w77] -> w63
          frame False {
          }
          frame True {
            n15 = Reverse 1D Array(array=w80) -> (reversed array=w79:cluster{"Output":dbl[], "Pwr out":dbl[]}[])
            n16 = Reverse 1D Array(array=w78) -> (reversed array=w77:string[])
          }
        }
        n17 = Select(t=u8 1 ("Y Scale.Mapping Mode"), s=w62, f=u8 0) -> (s? t:f=w59:u8)
        n18 = property on="XY Graph" class="XYGraph (strict)"("Y Scale.Mapping Mode"=w59) -> ()  [unwired: 2 in, 2 out]
        n19 = Array Size(array=w64) -> (size(s)=→"No of Series":i32)
        n20 = Build Path(base path="Job Directory", name or relative path="gnuplots") -> (appended path=w71:path)
      }
      frame "Fill label options" {
        n21 = Index Array(array=w94, index (col)=0 ("disabled index (col)")) -> (element=w82:string[])  [unwired: 1 in]
        n22 = Build Array (concatenate)("Title String Only", w82) -> (w81:string[])
        n23 = Build Array (concatenate)("All Series", w86) -> (w87:string[])
        n24 = property on="Added labels" class="LstBox (strict)"("Item Names"=w82) -> ()  [unwired: 2 in, 2 out]
        n25 = property on="Plot Title" class="Ring (strict)"("Strings []"=w81) -> ()  [unwired: 2 in, 2 out]
        n26 = property on="Ring" class="Ring (strict)"("Strings []"=w84) -> ()  [unwired: 2 in, 2 out]
        n27 = property on="Summarise" class="Ring (strict)"("Strings []"=w87) -> ()  [unwired: 2 in, 2 out]
      }
      frame "Sort plot points" {
        n28 = Equal?(x=w100, y=w101) -> (x = y?=w105:bool)
        n29 = for {
          tunnel: w104 -> [w127] mode=indexing
          tunnel: [w128] -> w103 mode=indexing
          tunnel: w105 -> [w121]
          n30 = Unbundle(w127) -> ("Output"=w126:dbl[], "Pwr out"=w123:dbl[])
          n31 = case shown="False" w121 {
            tunnel: [w145 w147] -> w120
            tunnel: w126 -> [w144 w147]
            tunnel: w123 -> [w145 w146]
            tunnel: [w144 w146] -> w122
            frame False {
            }
            frame True {
            }
          }
          n32 = Sort 1D Array(array=w120) -> (sorted array=w118:dbl[])
          n33 = for {
            tunnel: w120 -> [w139]
            tunnel: w118 -> [w135] mode=indexing
            tunnel: w122 -> [w138]
            tunnel: [w137] -> w117 mode=indexing
            shift-right: [w129] -> _
            shift-left: 0 ("f") -> [w132]
            shift-right: [w135] -> _
            shift-left: _ -> [w136]
            n34 = Equal?(x=w135, y=w136) -> (x = y?=w133:bool)
            n35 = Select(t=w132, s=w133, f=0) -> (s? t:f=w130:i32)
            n36 = Search 1D Array(1D array=w139, element=w135, start index (0)=w130) -> (index of element=w134:i32)
            n37 = Increment(x=w134) -> (x+1=w129:i32)
            n38 = Index Array(array=w138, index=w134) -> (element=w137:dbl)
          }
          n39 = call "Remove_duplicated_XY_val.vi"("Y values"=w117, "Sorted X values"=w118) -> ("Y Out"=w115:dbl[], "X out"=w116:dbl[])
          n40 = case shown="False" w121 {
            tunnel: [w140 w143] -> w125
            tunnel: w116 -> [w141 w143]
            tunnel: [w141 w142] -> w124
            tunnel: w115 -> [w140 w142]
            frame False {
            }
            frame True {
            }
          }
          n41 = Bundle("X out"=w125, "Y Out"=w124) -> (w128:cluster{"X out":dbl[], "Y Out":dbl[]})  [unwired: 1 in]
        }
        n42 = case shown="\"Spectrum\"" w97 {
          tunnel: ["Do fitting?" "Calculate % change" "Calculate Spectrum" "Calculate Normalised Spectrum"] -> w96
          tunnel: [FALSE ("Save data analysis file") FALSE ("Save data analysis file") TRUE ("Save data analysis file") TRUE ("Save data analysis file")] -> w95
          frame "None", Default {
          }
          frame "% change" {
          }
          frame "Spectrum" {
          }
          frame "Norm Spec" {
          }
        }
        n43 = local write "Save data analysis file"(w95) -> ()
      }
      frame "Calculate % change" {
        n44 = for {
          tunnel: w151 -> [w163] mode=indexing
          tunnel: [w155] -> w150 mode=indexing
          n45 = Unbundle(w163) -> ("Output"=w157:dbl[], "Pwr out"=w162:dbl[])
          n46 = call <vilib>:"Mean.vi"("X"=w162) -> ("mean"=w160:dbl)  [unwired: 1 out]
          n47 = Subtract(x=w162, y=w160) -> (x-y=w161:dbl[])
          n48 = Divide(x=w161, y=w160) -> (x/y=w159:dbl[])
          n49 = Multiply(x=w159, y=100.0) -> (x*y=w156:dbl[])
          n50 = Bundle("Output"=w157, w156) -> (w155:cluster{"Output":dbl[], dbl[]})  [unwired: 1 in]
        }
      }
      frame "Calculate Spectrum" {
        n51 = for {
          tunnel: w170 -> [w179] mode=indexing
          tunnel: [w180] -> w169 mode=indexing
          tunnel: [w175] -> w167 mode=indexing
          tunnel: w165 -> [w174] mode=indexing
          tunnel: [w173] -> w164 mode=indexing
          i -> [w176]
          n52 = Unbundle(w179) -> ("Output"=w177:dbl[], "Pwr out"=w178:dbl[])
          n53 = stacked-sequence {
            seq-local: [w182 _ _ _] -> [_ _ w225 _]
            seq-local: [w181 _ _ _] -> [_ w199 _ _]
            seq-local: [_ _ w221 _] -> [_ _ _ w256]
            seq-local: [_ _ w217 _] -> [_ _ _ w257]
            tunnel: [_ _ w232 _] -> w180
            tunnel: w178 -> [_ _ w219 _]
            tunnel: w177 -> [w193 _ w213 _]
            tunnel: w176 -> [_ w200 _ _]
            tunnel: [_ w199 _ _] -> w175
            tunnel: w174 -> [_ _ _ w252]
            tunnel: [_ _ _ w250] -> w173
            frame #0 {
              n54 = Index Array(array=w193, index=0) -> (element=w192:dbl)
              n55 = Array Subset(array=w193, index=1) -> (w191:dbl[])  [unwired: 1 in]
              n56 = for {
                shift-right: [w197] -> _
                shift-left: w192 -> [w198]
                tunnel: w191 -> [w197] mode=indexing
                tunnel: [w196] -> w188 mode=indexing
                n57 = Subtract(x=w197, y=w198) -> (x-y=w196:dbl)
              }
              n58 = call <vilib>:"Mean.vi"("X"=w188) -> ("mean"=w182:dbl)  [unwired: 1 out]
              n59 = Array Max & Min(array=w188) -> (max value=w190:dbl, min value=w189:dbl)  [unwired: 2 out]
              n60 = Absolute Value(x=w182) -> (abs(x)=w185:dbl)
              n61 = Subtract(x=w190, y=w189) -> (x-y=w187:dbl)
              n62 = Divide(x=w185, y=95.0) -> (x/y=w183:dbl)
              n63 = Absolute Value(x=w187) -> (abs(x)=w186:dbl)
              n64 = Less?(x=w186, y=w183) -> (x < y?=w181:bool)
            }
            frame #1 {
              n65 = case shown="False" w199 {
                tunnel: w200 -> [w205 _]
                frame False {
                  n66 = Increment(x=w205) -> (x+1=w204:i32)
                  n67 = Format Into String(format string="The positions are not evenly spaced so cannot calculate the spectrum for series %d", w204) -> (resulting string=w202:string)  [unwired: 2 in, 1 out]
                  n68 = One Button Dialog(message=w202, button name ("OK")="stop") -> ()  [unwired: 1 out]
                }
                frame True {
                }
              }
            }
            frame #2 {
              n69 = Reciprocal(x=w225) -> (1/x=w227:dbl)
              n70 = Array Size(array=w219) -> (size(s)=w226:i32)
              n71 = Divide(x=w227, y=w226) -> (x/y=w224:dbl)
              n72 = Divide(x=w224, y="DF Factor") -> (x/y=w222:dbl)
              n73 = Array Max & Min(array=w213) -> (max value=w212:dbl, min value=w211:dbl)  [unwired: 2 out]
              n74 = Subtract(x=w212, y=w211) -> (x-y=w210:dbl)
              n75 = Reciprocal(x=w210) -> (1/x=w209:dbl)
              n76 = Multiply(x=w209, y="Fmin Factor") -> (x*y=w208:dbl)
              n77 = call "DFT.vi"("dt"=w225, "Input Y"=w219, "Input X"=w213, "df"=w222, "fmin"=w208, "fmax"="fmax", "Windowing"="Window Type", "Autocorrelation before DFT"="Autocorrelation before DFT", "Mean shifting"="Mean shifting") -> ("Pwr out"=w218:dbl[], "Input to DFT"=w216:dbl[], "Actual fmin"=w228:dbl)  [unwired: 2 in, 2 out]
              n78 = case shown="False" "Case Constant\n(See Context Help)" {
                tunnel: w218 -> [w233 w238]
                tunnel: [w233 w237] -> w217
                tunnel: w216 -> [_ w236]
                frame False {
                }
                frame True {
                  n79 = call <vilib>:"Std Deviation and Variance.vi"("X"=w236, "Weighting (Sample)"=enum16{"Sample", "Population"}."Population") -> ("variance"=w234:dbl)  [unwired: 2 out]
                  n80 = Divide(x=w238, y=w234) -> (x/y=w237:dbl[])
                }
              }
              n81 = Array Size(array=w217) -> (size(s)=w231:i32)
              n82 = for {
                N: w231 -> [_]
                tunnel: [w245] -> w221 mode=indexing
                tunnel: w222 -> [w243]
                tunnel: w228 -> [w241]
                tunnel: "Freq?" -> [w239]
                i -> [w244]
                n83 = Multiply(x=w244, y=w243) -> (x*y=w242:dbl)
                n84 = Add(x=w242, y=w241) -> (x+y=w240:dbl)
                n85 = case shown="False" w239 {
                  tunnel: [w247 w248] -> w245
                  tunnel: w240 -> [w246 w248]
                  frame False {
                    n86 = Reciprocal(x=w246) -> (1/x=w247:dbl)
                  }
                  frame True {
                  }
                }
              }
              n87 = Bundle(w221, "Pwr out"=w217) -> (w232:cluster{dbl[], "Pwr out":dbl[]})  [unwired: 1 in]
            }
            frame #3 {
              n88 = Multiply(x=w256, y=w257) -> (x*y=w255:dbl[])
              n89 = Add Array Elements(numeric array=w257) -> (sum=w253:dbl)
              n90 = Add Array Elements(numeric array=w255) -> (sum=w254:dbl)
              n91 = Divide(x=w254, y=w253) -> (x/y=w251:dbl)
              n92 = case shown="True" "Wavelenght?" {
                tunnel: w252 -> [w258 w262]
                tunnel: w251 -> [_ w261]
                tunnel: [w258 w259] -> w250
                frame False {
                }
                frame True {
                  n93 = Format Into String(format string="Av Wavelength = %.1f; ", initial string=w262, w261) -> (resulting string=w259:string)  [unwired: 1 in, 1 out]
                }
              }
            }
          }
        }
        n94 = And Array Elements(Boolean array=w167) -> (logical AND=w166:bool)
      }
      frame "Calculate Normalised Spectrum" {
        n95 = for {
          tunnel: w268 -> [w275] mode=indexing
          tunnel: [w276] -> w267 mode=indexing
          tunnel: [w271] -> w264 mode=indexing
          i -> [w272]
          n96 = Unbundle(w275) -> ("Output"=w273:dbl[], "Pwr out"=w274:dbl[])
          n97 = stacked-sequence {
            seq-local: [w278 _ _] -> [_ _ w311]
            seq-local: [w277 _ _] -> [_ w295 _]
            tunnel: [_ _ w317] -> w276
            tunnel: w274 -> [_ _ w309]
            tunnel: w273 -> [w289 _ _]
            tunnel: w272 -> [_ w296 _]
            tunnel: [_ w295 _] -> w271
            frame #0 {
              n98 = Index Array(array=w289, index=0) -> (element=w288:dbl)
              n99 = Array Subset(array=w289, index=1) -> (w287:dbl[])  [unwired: 1 in]
              n100 = for {
                shift-right: [w293] -> _
                shift-left: w288 -> [w294]
                tunnel: w287 -> [w293] mode=indexing
                tunnel: [w292] -> w284 mode=indexing
                n101 = Subtract(x=w293, y=w294) -> (x-y=w292:dbl)
              }
              n102 = call <vilib>:"Mean.vi"("X"=w284) -> ("mean"=w278:dbl)  [unwired: 1 out]
              n103 = Array Max & Min(array=w284) -> (max value=w286:dbl, min value=w285:dbl)  [unwired: 2 out]
              n104 = Absolute Value(x=w278) -> (abs(x)=w281:dbl)
              n105 = Subtract(x=w286, y=w285) -> (x-y=w283:dbl)
              n106 = Divide(x=w281, y=95.0) -> (x/y=w279:dbl)
              n107 = Absolute Value(x=w283) -> (abs(x)=w282:dbl)
              n108 = Less?(x=w282, y=w279) -> (x < y?=w277:bool)
            }
            frame #1 {
              n109 = case shown="False" w295 {
                tunnel: w296 -> [w301 _]
                frame False {
                  n110 = Increment(x=w301) -> (x+1=w300:i32)
                  n111 = Format Into String(format string="The positions are not evenly spaced so cannot calculate the spectrum for series %d", w300) -> (resulting string=w298:string)  [unwired: 2 in, 1 out]
                  n112 = One Button Dialog(message=w298, button name ("OK")="stop") -> ()  [unwired: 1 out]
                }
                frame True {
                }
              }
            }
            frame #2 {
              w312 = 2 ("index")
              n113 = Reciprocal(x=w311) -> (1/x=w310:dbl)
              n114 = Array Size(array=w309) -> (size(s)=w313:i32)
              n115 = Divide(x=w310, y=w313) -> (x/y=w304:dbl)
              n116 = call "Power_spectrum.vi"("U"=w309, "Sampling frequency"=w310, "Block No"=1) -> ("Spectrum output array"=w307:dbl[])  [unwired: 3 in]
              n117 = call <vilib>:"Std Deviation and Variance.vi"("X"=w309) -> ("variance"=w308:dbl)  [unwired: 1 in, 2 out]
              n118 = Array Subset(array=w307, index=w312) -> (w303:dbl[])  [unwired: 1 in]
              n119 = Divide(x=w307, y=w308) -> (x/y=w306:dbl[])
              n120 = Divide(x=w303, y=w308) -> (x/y=w302:dbl[])
              n121 = Array Size(array=w302) -> (size(s)=w316:i32)
              n122 = for {
                N: w316 -> [_]
                tunnel: [w321] -> w315 mode=indexing
                tunnel: w304 -> [w323]
                tunnel: w312 -> [w319]
                i -> [w324]
                n123 = Increment(x=w324) -> (x+1=w320:i32)
                n124 = Add(x=w320, y=w319) -> (x+y=w318:i32)
                n125 = Multiply(x=w318, y=w323) -> (x*y=w322:dbl)
                n126 = Reciprocal(x=w322) -> (1/x=w321:dbl)
              }
              n127 = Bundle(w315, w302) -> (w317:cluster{dbl[], dbl[]})  [unwired: 1 in]
              n128 = Add Array Elements(numeric array=w306) -> (sum=w305:dbl)
              n129 = Multiply(x=w305, y=w304) -> ()  [unwired: 1 out]
            }
          }
        }
        n130 = And Array Elements(Boolean array=w264) -> (logical AND=w263:bool)
      }
      frame "Do fitting?" {
        n131 = case shown="\"Linear\", Default" w327 {
          tunnel: ["Adjust Plot scales etc" "Poly fit to data"] -> _
          frame "None" {
          }
          frame "Linear", Default {
          }
        }
      }
      frame "Poly fit to data" {
        n132 = case shown="\"None\", Default" w343 {
          tunnel: [0 ("polynomial order") 1 ("polynomial order") 2 ("polynomial order") 3 ("polynomial order") 4 ("polynomial order")] -> w342
          frame "None", Default {
          }
          frame "Linear" {
          }
          frame "2nd Ploy" {
          }
          frame "3rd Poly" {
          }
          frame "4th Poly" {
          }
        }
        n133 = for {
          tunnel: w341 -> [w365] mode=indexing
          tunnel: [w366] -> w340 mode=indexing
          tunnel: w342 -> [w364]
          tunnel: [w359] -> w337 mode=indexing
          tunnel: w336 -> [w358]
          tunnel: w335 -> [w357]
          w363 = 8  # Enhancement factor
          n134 = Unbundle(w365) -> ("Output"=w356:dbl[], "Pwr out"=w355:dbl[])
          n135 = call <vilib>:"General Polynomial Fit.vi"("Y"=w355, "polynomial order"=w364, "X"=w356) -> ("Polynomial Coefficients"=w353:dbl[])  [unwired: 9 in, 3 out]
          n136 = case shown="False" "Case Constant\n(See Context Help) 2" {
            tunnel: [w369 w384] -> w360
            tunnel: [w380 w385] -> w359
            tunnel: w358 -> [w382 _]
            tunnel: w357 -> [w381 _]
            tunnel: w356 -> [w377 _]
            tunnel: w355 -> [w374 _]
            tunnel: w353 -> [_ w384]
            frame False {
              w376 = 0.99 ("Voltage")
              n137 = Build Array (concatenate)(w376, w377) -> (w379:dbl[])
              n138 = Build Array (concatenate)(nan ("Voltage"), w374) -> (w378:dbl[])
              n139 = call "Curve_Fit_ph.vi"("Values In"=w378, "No of points to fit (3)"=4, "Positions"=w379) -> ("Values Out"=w373:dbl[], "Polynomial Fit Coefficients"=w369:dbl[])
              n140 = Index Array(array=w373, index=0) -> (element=w371:dbl)
              n141 = call "Number_2_string.vi"("precision"="2", "number"=w371) -> ("String"=w367:string)
              n142 = Format Into String(format string="When %s=%.2f ; %s=%s", w382, w376, w381, w367) -> (resulting string=w380:string)  [unwired: 2 in, 1 out]
            }
            frame True {
              n143 = for {
                shift-right: [w387] -> w385
                shift-left: "" -> [w388]
                tunnel: w384 -> [w391] mode=indexing
                i -> [w392]
                n144 = call "Number_2_string.vi"("number"=w391) -> ("String"=w389:string)  [unwired: 1 in]
                n145 = case shown="0, Default" w392 {
                  tunnel: [w393] -> w390
                  tunnel: w389 -> [w395]
                  frame 0, Default {
                    n146 = Concatenate Strings(w395, " ") -> (w393:string)
                  }
                }
                n147 = Concatenate Strings(w388, w390) -> (w387:string)
              }
            }
          }
          n148 = call "Enhance_No_of_points.vi"("Enhancement factor"=w363, "Input"=w356) -> ("Output"=w362:dbl[])  [unwired: 3 in]
          n149 = for {
            tunnel: w360 -> [w398]
            tunnel: w362 -> [w397] mode=indexing
            tunnel: [w396] -> w361 mode=indexing
            n150 = call "Polynomial_convert.vi"("Calib constants"=w398, "Voltage"=w397) -> ("Eng Values"=w396:dbl)  [unwired: 4 in]
          }
          n151 = Bundle("Output"=w362, w361) -> (w366:cluster{"Output":dbl[], dbl[]})  [unwired: 1 in]
        }
        n152 = Build Array (concatenate)(w339, w337) -> (w338:string[])
        n153 = Build Array (concatenate)(w341, w340) -> (w334:cluster{"Output":dbl[], "Pwr out":dbl[]}[])
        n154 = local write "XY Graph"(w334) -> ()
      }
      frame "Add fitted line styles" {
        n155 = local read "No of Series"() -> (w399:i32)
        n156 = Array Subset(array=w402, index=w399) -> (w401:string[])  [unwired: 1 in]
        n157 = for {
          tunnel: w401 -> [w410] mode=indexing
          tunnel: u8 2 ("Plot.Plot Interpolation") -> [w416]
          tunnel: w399 -> [w412]
          i -> [w413]
          w418 = u32 0
          n158 = Concatenate Strings(w410, "  " ("string")) -> (w408:string)
          n159 = Add(x=w412, y=w413) -> (x+y=w411:i32)
          n160 = Quotient & Remainder(x=w413, y=4) -> (x-y*floor(x/y)=w414:i32)  [unwired: 1 out]
          n161 = property on="XY Graph" class="XYGraph (strict)"("Active Plot"=w411, "Plot.Plot Name"=w408, "Plot.Fill/Point Color"=w418, "Plot.Plot Color"=w418, "Plot.Point Style"=u8 0, "Plot.Line Style"=w414, "Plot.Plot Interpolation"=w416) -> ()  [unwired: 2 in, 2 out]
        }
      }
      frame "Adjust Plot scales etc" {
        n162 = Greater Than 0?(x=w424) -> (x > 0?=w423:bool)
        n163 = Array Size(array=w426) -> (size(s)=w442:i32)
        n164 = property on="XY Graph" class="XYGraph (strict)"("Legend:Plots Shown"=w442) -> ()  [unwired: 2 in, 2 out]
        n165 = Build Array(u8 6 ("Write Attribute"), u8 1 ("Write Attribute"), u8 11 ("Write Attribute"), u8 2 ("Write Attribute"), u8 5 ("Write Attribute"), u8 13 ("Write Attribute"), u8 15 ("Write Attribute"), u8 10 ("Write Attribute"), u8 12 ("Write Attribute"), u8 14 ("Write Attribute")) -> (w430:u8[])
        n166 = local read "No of Series"() -> (w425:i32)
        n167 = case shown="\"None\", Default" w421 {
          tunnel: ["Adjust plot scales2" "Show percentage change" ("t") "Set spectra axis" ("t") "Set spectra axis" ("t")] -> w420
          frame "None", Default {
          }
          frame "% change" {
          }
          frame "Spectrum" {
          }
          frame "Norm Spec" {
          }
        }
        n168 = Select(t=u8 2 ("Plot.Plot Interpolation"), s=w423, f=u8 0 ("Plot.Plot Interpolation")) -> (s? t:f=w427:u8)
        n169 = for {
          N: w425 -> [_]
          tunnel: w426 -> [w456] mode=indexing
          tunnel: w430 -> [w460]
          tunnel: w427 -> [w449]
          i -> [w459]
          w461 = u32 0
          n170 = String Length(string=w456) -> (length=w452:i32)
          n171 = Subtract(x=w452, y=2) -> (x-y=w450:i32)
          n172 = String Subset(string=w456, offset (0)=0, length (rest)=w450) -> (substring=w455:string)
          n173 = Concatenate Strings(w455, "  " ("string")) -> (w453:string)
          n174 = Index Array(array=w460, index=w459) -> (element=w458:u8)
          n175 = property on="XY Graph" class="XYGraph (strict)"("Active Plot"=w459, "Plot.Plot Name"=w453, "Plot.Fill/Point Color"=w461, "Plot.Plot Color"=w461, "Plot.Point Style"=w458, "Plot.Line Style"=u8 0, "Plot.Plot Interpolation"=w449) -> ()  [unwired: 2 in, 2 out]
        }
        "XY Graph" <- w419
      }
      frame "Adjust plot scales2" {
        n176 = property on="XY Graph" class="XYGraph (strict)"("X Scale.Name Label.Text"=w466, "Y Scale.Name Label.Text"=w462, "Cursor.Visible"=FALSE) -> ()  [unwired: 2 in, 2 out]
      }
      frame "Show percentage change" {
        n177 = Concatenate Strings(w474, " % Change" ("string")) -> (w477:string)
        n178 = property on="XY Graph" class="XYGraph (strict)"("X Scale.Name Label.Text"=w475, "Y Scale.Name Label.Text"=w477, "Cursor.Visible"=FALSE) -> ()  [unwired: 2 in, 2 out]
      }
      frame "Set spectra axis" {
        n179 = case shown="\"Spectrum\", Default" w482 {
          tunnel: [" Spectral Energy" ("string") " Normalised Spectral Energy" ("string")] -> w490
          frame "Spectrum", Default {
          }
          frame "Norm Spec" {
          }
        }
        n180 = Concatenate Strings(w487, w490) -> (w489:string)
        n181 = property on="XY Graph" class="XYGraph (strict)"("X Scale.Name Label.Text"="Wavelength [mm]", "Y Scale.Name Label.Text"=w489, "Cursor.Visible"=FALSE) -> ()  [unwired: 2 in, 2 out]
      }
      frame "Fill Second legend" {
        n182 = stacked-sequence {
          seq-local: [_ w532 _ _ _] -> [_ _ w569 _ _]
          seq-local: [_ _ _ w588 _] -> [_ _ _ _ _]
          seq-local: [w507 _ _ _ _] -> [_ w531 _ _ _]
          seq-local: [_ _ _ w585 _] -> [_ _ _ _ _]
          tunnel: [_ "Sort out plot title" _ _ _] -> w504
          tunnel: [_ "Save Automatically?" _ _ _] -> w503
          tunnel: w502 -> [w510 w533 _ _ _]
          tunnel: w501 -> [_ _ _ _ _]
          tunnel: [_ _ _ _ w603] -> w500
          tunnel: w497 -> [w506 _ _ _ _]
          tunnel: w496 -> [_ _ _ _ w597]
          frame #0 {
            n183 = Index Array(array=w510, index (col)=0 ("disabled index (col)")) -> (element=w516:string[])  [unwired: 1 in]
            n184 = local read "No of Series"() -> (w505:i32)
            n185 = Search 1D Array(1D array=w516, element="Original:Results:Filename") -> (index of element=w515:i32)  [unwired: 1 in]
            n186 = Array Size(array=w506) -> ()  [unwired: 1 out]
            n187 = for {
              N: w505 -> [_]
              tunnel: w515 -> [w522]
              tunnel: w510 -> [w521]
              tunnel: [w519] -> w511 mode=indexing
              i -> [w524]
              n188 = Add(x=3, y=w524) -> (x+y=w520:i32)
              n189 = Index Array(array=w521, index (row)=w522, index (col)=w520) -> (element=w519:string)
            }
            n190 = call "Analyse_string_array.vi"("String array"=w511) -> ("Unique strings"=w512:string[])  [unwired: 1 in, 1 out]
            n191 = Array Size(array=w512) -> (size(s)=w514:i32)
            n192 = Equal?(x=w514, y=1) -> (x = y?=w509:bool)
            n193 = Select(t=1, s=w509, f=w505) -> (s? t:f=w507:i32)
          }
          frame #1 {
            (unwired) "Date:of:Measurement"
            n194 = Index Array(array=w533, index (col)=0 ("disabled index (col)")) -> (element=w541:string[])  [unwired: 1 in]
            n195 = Equal?(x=w531, y=1) -> (x = y?=w529:bool)
            n196 = Search 1D Array(1D array=w541, element="Current:Data:Filename") -> (index of element=w536:i32)  [unwired: 1 in]
            "Current filename index" <- w536
            n197 = Select(t=2, s=w529, f=3 ("disabled index (col)")) -> (s? t:f=w527:i32)
            n198 = Search 1D Array(1D array=w541, element="Seconds:Since:1904") -> (index of element=w540:i32)  [unwired: 1 in]
            n199 = Search 1D Array(1D array=w541, element="Original:Results:Filename") -> (index of element=w537:i32)  [unwired: 1 in]
            n200 = for {
              N: w531 -> [_]
              tunnel: w540 -> [w557]
              tunnel: w537 -> [w556]
              tunnel: w536 -> [w555]
              tunnel: w533 -> [w554]
              tunnel: [w552] -> w532 mode=indexing
              tunnel: w527 -> [w548]
              i -> [w551]
              n201 = Add(x=w548, y=w551) -> (x+y=w553:i32)
              n202 = Index Array(array=w554, index (col)=w553) -> (element=w558:string[])  [unwired: 1 in]
              n203 = Index Array(array=w558, index=w555) -> (element=w547:string)
              n204 = Index Array(array=w558, index=w557) -> (element=w546:string)
              n205 = Index Array(array=w558, index=w556) -> (element=w550:string)
              n206 = Equal?(x=w547, y=w550) -> (x = y?=w549:bool)
              n207 = call "Display_data_dates.vi"("String"=w546) -> ("resulting string"=w545:string)
              n208 = Concatenate Strings("    " ("string"), w545) -> (w543:string)
              n209 = case shown="False" w549 {
                tunnel: [w561 w566] -> w552
                tunnel: w547 -> [w560 w563]
                tunnel: w550 -> [_ w564]
                tunnel: w543 -> [w559 w565]
                frame True {
                  n210 = Format Into String(format string="%s; %s", w560, w559) -> (resulting string=w561:string)  [unwired: 2 in, 1 out]
                }
                frame False {
                  n211 = Format Into String(format string="Cur  %s; Orig  %s; %s", w563, w564, w565) -> (resulting string=w566:string)  [unwired: 2 in, 1 out]
                }
              }
            }
          }
          frame #2 {
            n212 = call "Analyse_string_array.vi"("String array"=w569) -> ("Unique strings"=w570:string[])  [unwired: 1 in, 1 out]
            n213 = Array Size(array=w570) -> (size(s)=w574:i32)
            n214 = Equal?(x=w574, y=1) -> (x = y?=w572:bool)
            n215 = case shown="False" w572 {
              tunnel: w570 -> [_ w584]
              tunnel: [w577 w584] -> w568
              tunnel: [w575 1] -> _
              tunnel: w569 -> [w576 _]
              frame False {
                n216 = for {
                  tunnel: w576 -> [w580] mode=indexing
                  tunnel: [w578] -> w577 mode=indexing
                  i -> [w582]
                  n217 = Increment(x=w582) -> (x+1=w581:i32)
                  n218 = Format Into String(format string="Series %d; %s", w581, w580) -> (resulting string=w578:string)  [unwired: 2 in, 1 out]
                }
                n219 = Array Size(array=w576) -> (size(s)=w575:i32)
              }
              frame True {
              }
            }
            n220 = Build Array(w568) -> (w571:string[][])
            n221 = Transpose 2D Array(2D array=w571) -> ()  [unwired: 1 out]
          }
          frame #3 {
            n222 = property on="XY Graph" class="XYGraph (strict)" props=["Legend:Position:Top", "Legend:Size:Height", "Legend:Plots Shown"]() -> ("Legend:Position:Top"=w585:i32, "Legend:Size:Height"=w587:u32)  [unwired: 2 in, 3 out]
            n223 = Add(x=w585, y=w587) -> (x+y=w590:u32)
            n224 = To Long Integer(number=w590) -> (32bit integer=w586:i32)
            n225 = Add(x=w586, y=28) -> (x+y=w588:i32)
          }
          frame #4 {
            n226 = global read "Results_plotter_Global.vi" "Current Data Filenames"() -> (w593:string)
            n227 = call "Fast_string_Replace.vi"("Replace match with:"="_", "Input String"=w593, "regular expression"="[/]") -> ("Output String"=w598:string)  [unwired: 1 in, 1 out]
            n228 = call "Fast_string_Replace.vi"("Replace match with:"="_", "Input String"=w598, "regular expression"="__") -> ("Output String"=w594:string)  [unwired: 1 in, 1 out]
            n229 = call "Fast_string_Replace.vi"("Replace match with:"="", "Input String"=w594, "regular expression"=" ") -> ("Output String"=w592:string)  [unwired: 1 in, 1 out]
            n230 = String Subset(string=w592, offset (0)=0, length (rest)=30 ("length (rest)")) -> (substring=w591:string)
            n231 = Build Path(base path=w597, name or relative path=w591) -> (appended path=w603:path)
          }
        }
      }
      frame "Sort out plot title" {
        n232 = local read "Summarise"() -> (w610:u16)
        n233 = case shown="1, Default" "Plot Title" {
          tunnel: [w617 w623] -> w606
          tunnel: "Plot Title" -> [w617 w622]
          tunnel: w611 -> [_ w627]
          tunnel: "Plot Title" -> [_ w626]
          tunnel: w610 -> [_ w620]
          frame 0 {
          }
          frame 1, Default {
            n234 = Decrement(x=w626) -> (x-1=w625:u16)
            n235 = Add(x=w620, y=u16 2) -> (x+y=w619:u16)
            n236 = Index Array(array=w627, index (row)=w625, index (col)=w619) -> (element=w630:string)
            n237 = Empty String/Path?(string/path=w622) -> (empty?=w624:bool)
            n238 = call "Fast_string_Replace.vi"("Replace match with:"="~ ", "Input String"=w630, "regular expression"=":") -> ("Output String"=w629:string)  [unwired: 1 in, 1 out]
            n239 = call <vilib>:"Trim Whitespace.vi"("string"=w629) -> ("trimmed string"=w628:string)  [unwired: 1 in]
            n240 = call "Fast_string_Replace.vi"("Replace match with:"="~", "Input String"=w628, "regular expression"="_") -> ("Output String"=w618:string)  [unwired: 1 in, 1 out]
            n241 = case shown="False" w624 {
              tunnel: [w636 w639] -> w623
              tunnel: w618 -> [w638 w639]
              tunnel: w622 -> [w637 _]
              frame False {
                n242 = Concatenate Strings(w637, " " ("string"), w638) -> (w636:string)
              }
              frame True {
              }
            }
          }
        }
        "Final Title" <- w606
      }
      frame "Get Filename" {
        n243 = local read "Final Title"() -> (w643:string)
        n244 = case shown="\"% change\"" w646 {
          tunnel: ["" "Per_" "Spec_" "N_Spec_"] -> w644
          frame "None" {
          }
          frame "% change" {
          }
          frame "Spectrum" {
          }
          frame "Norm Spec" {
          }
        }
        n245 = String Length(string=w643) -> (length=w642:i32)
        n246 = Concatenate Strings(w644, w643) -> (w640:string)
        n247 = case shown="1, Default" w642 {
          tunnel: [w661 w662] -> w641
          tunnel: w640 -> [w661 w664]
          frame 0 {
          }
          frame 1, Default {
            n248 = Concatenate Strings(w664, "_") -> (w662:string)
          }
        }
        n249 = case shown="True" "Tweak scale" {
          frame False {
          }
          frame True {
            n250 = property on="XY Graph" class="XYGraph (strict)"("Y Scale.Range:Minimum"=0.0) -> ()  [unwired: 2 in, 2 out]
          }
        }
        n251 = call "Auto_filename.vi"("Filename Max length"="Filename Max length", "Prefix"=w641) -> ("Filename"=w648:string)
        n252 = Build Path(base path=w655, name or relative path=w648) -> (appended path=w652:path)
        n253 = Build Path(base path=w652, name or relative path=w648) -> (appended path=w659:path)
        n254 = File/Directory Info(path=w652) -> (error out=w653:errorcluster)  [unwired: 1 in, 6 out]
        n255 = Unbundle By Name(w653) -> ("status"=w651:bool)
        n256 = Select(t="Create plot directory", s=w651, f="Find a unique name") -> (s? t:f=w658:string)
      }
      frame "Find a unique name" {
        n257 = Strip Path(path=w677) -> (stripped path=w676:path, name=w675:string)
        n258 = Strip Path(path=w676) -> (stripped path=w673:path)  [unwired: 1 out]
        n259 = List Folder(path=w673) -> (folder names=w674:string[])  [unwired: 3 in, 3 out]
        n260 = while {
          tunnel: w675 -> [w698]
          tunnel: 27 ("Max Length") -> [w697]
          tunnel: [w686] -> w672
          tunnel: w674 -> [w687]
          i -> [w688]
          stop <- w684 continue-if-true
          n261 = Add(x=97, y=w688) -> (x+y=w695:i32)
          n262 = Build Array(w695) -> (w696:i32[])
          n263 = Byte Array To String(unsigned byte array=w696) -> (string=w693:string)
          n264 = Concatenate Strings(w698, w693) -> (w691:string)
          n265 = Reverse String(1:w691) -> (0:w692:string)
          n266 = String Subset(string=w692, offset (0)=0, length (rest)=w697) -> (substring=w690:string)
          n267 = Reverse String(1:w690) -> (0:w686:string)
          n268 = Search 1D Array(1D array=w687, element=w686) -> (index of element=w685:i32)  [unwired: 1 in]
          n269 = Greater Or Equal To 0?(x=w685) -> (x >= 0?=w684:bool)
        }
        n270 = Build Path(base path=w673, name or relative path=w672) -> (appended path=w671:path)
        n271 = Build Path(base path=w671, name or relative path=w672) -> (appended path=w670:path)
      }
      frame "Create plot directory" {
        n272 = call "Create_directory_path.vi"("Path name"=w704) -> ("Path name Out"=w703:path)
        n273 = Select(t="Save data analysis file", s="Save data analysis file", f="Save .dat file") -> (s? t:f=w701:string)
      }
      frame "Save data analysis file" {
        n274 = stacked-sequence {
          seq-local: [w722 _ _] -> [_ _ w766]
          seq-local: [_ w738 _] -> [_ _ w764]
          tunnel: w720 -> [_ _ w777]
          tunnel: [_ _ TRUE ("Top Level")] -> w719
          tunnel: [_ _ "Save .dat file"] -> w718
          tunnel: w717 -> [w725 w740 _]
          tunnel: w716 -> [_ _ _]
          tunnel: w715 -> [_ _ _]
          tunnel: w709 -> [_ w741 _]
          tunnel: w714 -> [_ _ _]
          tunnel: w713 -> [_ _ _]
          tunnel: w712 -> [_ _ _]
          tunnel: w711 -> [w729 _ _]
          tunnel: w710 -> [w728 _ _]
          frame #0 {
            n275 = case shown="\"Norm Spec\"" w729 {
              tunnel: w728 -> [w732 w736]
              tunnel: [w731 w735] -> w727
              tunnel: ["Wavelength::[mm]" "Wavelength::[mm]"] -> w726
              frame "Spectrum", Default {
                n276 = Concatenate Strings(w732, ":Spectral:Energy") -> (w731:string)
              }
              frame "Norm Spec" {
                n277 = Concatenate Strings(w736, ":Normalised Spectral:Energy") -> (w735:string)
              }
            }
            n278 = Index Array(array=w725, index (col)=0 ("disabled index (col)")) -> (element=w723:string[])  [unwired: 1 in]
            n279 = Build Array (concatenate)(w726, w727, w723) -> (w722:string[])
          }
          frame #1 {
            n280 = for {
              tunnel: w741 -> [w752] mode=indexing
              tunnel: w740 -> [w749]
              shift-right: [w743] -> w738
              shift-left: string[][] [] -> [w742]
              i -> [w747]
              n281 = Unbundle(w752) -> ("Output"=w751:dbl[], "Pwr out"=w750:dbl[])
              n282 = Add(x=3 ("disabled index (col)"), y=w747) -> (x+y=w746:i32)
              n283 = Index Array(array=w749, index (col)=w746) -> (element=w745:string[])  [unwired: 1 in]
              n284 = for {
                tunnel: w751 -> [w758] mode=indexing
                tunnel: w750 -> [w757] mode=indexing
                tunnel: w745 -> [w754]
                tunnel: [w753] -> w744 mode=indexing
                n285 = call "Number_2_string.vi"("number"=w758) -> ("String"=w756:string)  [unwired: 1 in]
                n286 = call "Number_2_string.vi"("number"=w757) -> ("String"=w755:string)  [unwired: 1 in]
                n287 = Build Array (concatenate)(w756, w755, w754) -> (w753:string[])
              }
              n288 = Build Array (concatenate)(w742, w744) -> (w743:string[][])
            }
          }
          frame #2 {
            w773 = FALSE  # Append last row only
            w772 = FALSE  # exists?
            n289 = Strip Path(path=w777) -> (stripped path=w778:path, name=w780:string)
            n290 = Array Size(array=w764) -> (size(s)=w763:i32[])
            n291 = Concatenate Strings(w780, ".xls" ("string")) -> (w779:string)
            n292 = Index Array(array=w763, index=0) -> (element=w761:i32)
            n293 = Build Path(base path=w778, name or relative path=w779) -> (appended path=w767:path)
            n294 = Initialize Array("", w761) -> (w760:string[])
            n295 = Build Array (concatenate)(w760, w764) -> (w765:string[][])
            n296 = Initialize Array("", 10 ("Dimension Size")) -> (w771:string[])
            n297 = call "Asterisk_header.vi"("Channel names"=w771) -> ("Header string"=w768:string)
            n298 = call "Write_Ch_data_file.vi"("Append last row only"=w773, "Header string"=w768, "exists?"=w772, "Channel Values"=w765, "Channel names"=w766, "Filename"=w767) -> ()  [unwired: 6 in]
          }
        }
      }
      frame "Save .dat file" {
        n299 = stacked-sequence {
          seq-local: [w795 _ _ _ _] -> [_ _ _ _ w881]
          seq-local: [_ w821 _ _ _] -> [_ _ _ _ w882]
          seq-local: [_ _ _ w841 _] -> [_ _ _ _ w883]
          seq-local: [_ _ w832 _ _] -> [_ _ _ w839 _]
          tunnel: w793 -> [_ _ _ _ w886]
          tunnel: [_ _ _ _ TRUE ("Top Level")] -> w792
          tunnel: [_ _ _ _ "Gnuplot script Start"] -> w791
          tunnel: w790 -> [w800 _ _ _ _]
          tunnel: w789 -> [_ w824 _ _ _]
          tunnel: w788 -> [_ w820 _ _ _]
          tunnel: w787 -> [_ _ _ w843 _]
          tunnel: w786 -> [_ _ _ w840 _]
          tunnel: w785 -> [_ _ _ _ _]
          tunnel: w784 -> [_ _ _ _ _]
          tunnel: w783 -> [_ w818 _ _ _]
          tunnel: [_ _ _ w838 _] -> w782
          tunnel: w781 -> [_ _ w830 _ _]
          frame #0 {
            n300 = Array Subset(array=w800, length (col)=3 ("length")) -> (w798:string[][])  [unwired: 3 in]
            n301 = Build Array("Column Name", "Numeric Tolerance", "Range of Values") -> (w804:string[])
            n302 = Build Array (concatenate)(w804, w798) -> (w796:string[][])
            n303 = for {
              shift-right: [w808] -> w795
              shift-left: "" -> [w805]
              tunnel: w796 -> [w809] mode=indexing
              n304 = for {
                shift-right: [w810] -> w807
                shift-left: w805 -> [w817]
                tunnel: w809 -> [w811] mode=indexing
                i -> [w816]
                n305 = Equal To 0?(x=w816) -> (x = 0?=w815:bool)
                n306 = Select(t="#", s=w815, f="\t") -> (s? t:f=w812:string)
                n307 = Concatenate Strings(w817, w812, w811) -> (w810:string)
              }
              n308 = Concatenate Strings(w807, "\n") -> (w808:string)
            }
          }
          frame #1 {
            w822 = "\n"
            n309 = case shown="\"% change\"" w818 {
              tunnel: w820 -> [w826 w828]
              tunnel: [w826 w827] -> w819
              frame "None", Default {
              }
              frame "% change" {
                n310 = Concatenate Strings(w828, " %" ("string")) -> (w827:string)
              }
            }
            n311 = Concatenate Strings(w822, w822, "#" ("string"), w824, "\t", w819, w822, w822) -> (w821:string)
          }
          frame #2 {
            n312 = case shown="True" "Offset?" {
              tunnel: [0.0 w835] -> w833
              frame False {
              }
              frame True {
                n313 = property on="XY Graph" class="XYGraph (strict)"() -> ("Y Scale.Range:Maximum"=w837:dbl, "Y Scale.Range:Minimum"=w836:dbl)  [unwired: 2 in, 2 out]
                n314 = Subtract(x=w837, y=w836) -> (x-y=w835:dbl)
              }
            }
            "Profile offset" <- w833
            n315 = Multiply(x=w833, y=w830) -> (x*y=w832:dbl)
          }
          frame #3 {
            n316 = for {
              tunnel: w843 -> [w865] mode=indexing
              shift-right: [w864] -> w841
              shift-left: "" -> [w856]
              tunnel: w840 -> [w854] mode=indexing
              tunnel: w839 -> [w851]
              tunnel: [w857] -> w838 mode=indexing
              i -> [w860]
              w863 = "\n"
              n317 = Unbundle(w865) -> ("Output"=w844:dbl[], "Pwr out"=w859:dbl[])
              n318 = Multiply(x=w851, y=w860) -> (x*y=w846:dbl)
              n319 = Negate(x=w846) -> (-x=w845:dbl)
              n320 = call "Number_2_string.vi"("number"=w845) -> ("String"=w853:string)  [unwired: 1 in]
              n321 = Format Into String(format string="\\t%s\\tPlot offset", w853) -> (resulting string=w849:string)  [unwired: 2 in, 1 out]
              n322 = for {
                tunnel: w844 -> [w875] mode=indexing
                shift-right: [w872] -> w862
                shift-left: "" -> [w874]
                tunnel: w863 -> [w869]
                tunnel: w859 -> [w868] mode=indexing
                tunnel: w846 -> [w867]
                tunnel: [w866] -> w858 mode=indexing
                n323 = Subtract(x=w868, y=w867) -> (x-y=w866:dbl)
                n324 = call "Number_2_string.vi"("number"=w875) -> ("String"=w873:string)  [unwired: 1 in]
                n325 = call "Number_2_string.vi"("number"=w866) -> ("String"=w871:string)  [unwired: 1 in]
                n326 = Concatenate Strings(w874, w873, "\t", w871, w869) -> (w872:string)
              }
              n327 = Equal To 0?(x=w846) -> (x = 0?=w850:bool)
              n328 = Select(t="", s=w850, f=w849) -> (s? t:f=w847:string)
              n329 = Concatenate Strings(w856, "#", w854, w847, w863, w862, w863, w863) -> (w864:string)
              n330 = Bundle("Output"=w844, w858) -> (w857:cluster{"Output":dbl[], dbl[]})  [unwired: 1 in]
            }
          }
          frame #4 {
            w878 = FALSE  # advisory dialog? (display:T)
            w879 = FALSE  # append to file? (new file:F)
            n331 = Strip Path(path=w886) -> (stripped path=w887:path, name=w889:string)
            n332 = Concatenate Strings(w881, w882, w883) -> (w880:string)
            n333 = Concatenate Strings(w889, ".dat" ("string")) -> (w888:string)
            n334 = Build Path(base path=w887, name or relative path=w888) -> (appended path=w877:path)
            n335 = call "Write_Characters_To_File.vi"("file path (dialog if empty)"=w877, "advisory dialog? (display:T)"=w878, "character string"=w880, "append to file? (new file:F)"=w879) -> ()  [unwired: 4 in, 1 out]
          }
        }
      }
      frame "Gnuplot script Start" {
        n336 = case shown="\"Norm Spec\"" w909 {
          tunnel: w908 -> [w919 w922 w926 w930]
          tunnel: [w919 w921 w925 w929] -> w905
          tunnel: [w918 w920 "Wavelength [mm]" ("X Axis Name") "Wavelength [mm]" ("X Axis Name")] -> w906
          tunnel: w907 -> [w918 w920 _ _]
          frame "None", Default {
          }
          frame "% change" {
            n337 = Concatenate Strings(w922, " % change" ("string")) -> (w921:string)
          }
          frame "Spectrum" {
            n338 = Concatenate Strings(w926, " Spectral energy" ("string")) -> (w925:string)
          }
          frame "Norm Spec" {
            n339 = Concatenate Strings(w930, " Normalised Spectral Energy" ("string")) -> (w929:string)
          }
        }
        n340 = local read "Final Title"() -> (w891:string)
        n341 = call "Text_for_latex.vi"("Input String"=w891) -> ("Output String"=w892:string)
        n342 = call "Text_for_latex.vi"("Input String"=w906) -> ("Output String"=w902:string)
        n343 = call "Text_for_latex.vi"("Input String"=w905) -> ("Output String"=w899:string)
        n344 = call "Fast_string_Replace.vi"("Replace match with:"="", "Input String"=w892, "regular expression"="[$]") -> ("Output String"=w890:string)  [unwired: 1 in, 1 out]
        n345 = call "Fast_string_Replace.vi"("Replace match with:"="", "Input String"=w902, "regular expression"="[$]") -> ("Output String"=w898:string)  [unwired: 1 in, 1 out]
        n346 = call "Fast_string_Replace.vi"("Replace match with:"="", "Input String"=w899, "regular expression"="[$]") -> ("Output String"=w897:string)  [unwired: 1 in, 1 out]
        n347 = Format Into String(format string="set term epslatex\\nset output \"Plot.eps\"\\nset xlabel '$%s$'\\nset ylabel '$%s$'\\nset samples 1000\\nset pointsize %.2f\\nset title '$%s$' 0, 0\\nset size %s,%s\n", w898, w897, "Point Size", w890, "Graph width", "Graph Height") -> (resulting string=w915:string)  [unwired: 2 in, 1 out]
      }
      frame "Edit Legend names" {
        n348 = local read "Profile offset"() -> (w935:dbl)
        n349 = Multiply(x=w937, y=w935) -> (x*y=w939:dbl)
        n350 = for {
          tunnel: w946 -> [w950] mode=indexing
          tunnel: [w948] -> w945 mode=indexing
          tunnel: [w947] -> w940
          i -> [w947]
          n351 = String Length(string=w950) -> (length=w953:i32)
          n352 = Subtract(x=w953, y=2) -> (x-y=w951:i32)
          n353 = String Subset(string=w950, length (rest)=w951) -> (substring=w949:string)  [unwired: 1 in]
          n354 = call "Text_for_latex.vi"("Input String"=w949) -> ("Output String"=w948:string)
        }
        n355 = Decrement(x=w937) -> (x-1=w936:dbl)
        n356 = Multiply(x=w939, y=w940) -> (x*y=w934:dbl)
        n357 = Multiply(x=w935, y=w936) -> (x*y=w933:dbl)
        n358 = Add(x=w933, y=w934) -> (x+y=→"Extra range":dbl)
      }
      frame "Input Legend info" {
        n359 = local read "Graph Height"() -> (w962:string)
        n360 = Array Size(array="Added labels") -> (size(s)=w973:i32)
        n361 = Fract/Exp String To Number(string=w962) -> (number=w961:dbl)  [unwired: 3 in, 1 out]
        n362 = case shown="False" w980 {
          tunnel: w988 -> [_ w1025]
          tunnel: [w1012 w1024] -> w968
          tunnel: [w1011 w1023] -> w964
          tunnel: [w1001 w1022] -> w987
          tunnel: [w1005 w1021] -> w986
          tunnel: [w1009 0.7 ("y")] -> w979
          tunnel: [0.9 ("y") 0.95 ("y")] -> w978
          tunnel: w961 -> [w1008 _]
          tunnel: w960 -> [_ _]
          tunnel: w959 -> [w1004 _]
          frame False {
            n363 = property on="XY Graph" class="XYGraph (strict)"() -> ("X Scale.Range:Maximum"=w1012:dbl, "X Scale.Range:Minimum"=w1011:dbl, "Y Scale.Range:Maximum"=w1003:dbl, "Y Scale.Range:Minimum"=w1002:dbl)  [unwired: 2 in, 2 out]
            n364 = local read "Extra range"() -> (w1006:dbl)
            n365 = case shown="True" w1004 {
              tunnel: w1003 -> [w1014 w1018]
              tunnel: w1002 -> [w1013 w1017]
              tunnel: [w1014 w1016] -> w1001
              tunnel: [w1013 w1015] -> w1000
              frame False {
              }
              frame True {
                n366 = Logarithm Base 10(1:w1018) -> (0:w1016:dbl)
                n367 = Logarithm Base 10(1:w1017) -> (0:w1015:dbl)
              }
            }
            n368 = Divide(x=0.35 ("y"), y=w1008) -> (x/y=w1009:dbl)
            n369 = Subtract(x=w1000, y=w1006) -> (x-y=w1005:dbl)
          }
          frame True {
            n370 = for {
              shift-right: [w1040] -> w1024
              shift-left: _ -> [w1032]
              shift-right: [w1034] -> w1021
              shift-left: _ -> [w1030]
              shift-right: [w1038] -> w1023
              shift-left: _ -> [w1029]
              shift-right: [w1036] -> w1022
              shift-left: _ -> [w1031]
              tunnel: w1025 -> [w1028] mode=indexing
              i -> [w1041]
              n371 = Unbundle(w1028) -> ("Output"=w1027:dbl[], "Pwr out"=w1026:dbl[])
              n372 = Array Max & Min(array=w1027) -> (max value=w1039:dbl, min value=w1037:dbl)  [unwired: 2 out]
              n373 = Array Max & Min(array=w1026) -> (max value=w1035:dbl, min value=w1033:dbl)  [unwired: 2 out]
              n374 = case shown="1, Default" w1041 {
                tunnel: [w1045 w1058] -> w1040
                tunnel: w1039 -> [w1045 w1060]
                tunnel: [w1044 w1046] -> w1038
                tunnel: w1037 -> [w1044 w1051]
                tunnel: [w1043 w1047] -> w1036
                tunnel: w1035 -> [w1043 w1054]
                tunnel: [w1042 w1048] -> w1034
                tunnel: w1033 -> [w1042 w1049]
                tunnel: w1032 -> [_ w1059]
                tunnel: w1031 -> [_ w1053]
                tunnel: w1030 -> [_ w1052]
                tunnel: w1029 -> [_ w1050]
                frame 0 {
                }
                frame 1, Default {
                  n375 = Greater?(x=w1060, y=w1059) -> (0:w1061:bool)
                  n376 = Less?(x=w1051, y=w1050) -> (x < y?=w1055:bool)
                  n377 = Greater?(x=w1054, y=w1053) -> (0:w1057:bool)
                  n378 = Less?(x=w1049, y=w1052) -> (x < y?=w1056:bool)
                  n379 = Select(t=w1060, s=w1061, f=w1059) -> (s? t:f=w1058:dbl)
                  n380 = Select(t=w1051, s=w1055, f=w1050) -> (s? t:f=w1046:dbl)
                  n381 = Select(t=w1054, s=w1057, f=w1053) -> (s? t:f=w1047:dbl)
                  n382 = Select(t=w1049, s=w1056, f=w1052) -> (s? t:f=w1048:dbl)
                }
              }
            }
          }
        }
        n383 = Greater Than 0?(x=w973) -> (x > 0?=w972:bool)
        n384 = Select(t="Add Labels to plot", s=w972, f="Set plot ranges" ("t")) -> (s? t:f=w969:string)
        n385 = Subtract(x=w968, y=w964) -> (x-y=w967:dbl)
        n386 = Subtract(x=w987, y=w986) -> (x-y=w977:dbl)
        n387 = Divide(x=w977, y=10.0) -> (x/y=w975:dbl)
        "Delta y" <- w975
        n388 = Multiply(x=-0.2, y=w967) -> (x*y=w965:dbl)
        n389 = Multiply(x=w967, y=w978) -> (x*y=w990:dbl)
        n390 = Multiply(x=w977, y=w979) -> (x*y=w989:dbl)
        n391 = Add(x=w964, y=w965) -> (x+y=→"X location":dbl)
        n392 = Add(x=w964, y=w990) -> (x+y=w957:dbl)
        n393 = Subtract(x=w986, y=w989) -> (x-y=w958:dbl)
        "Y location" <- w958
        n394 = case shown="True" "Show legend?" {
          tunnel: "" -> [w1064 w1073]
          tunnel: "#" -> [w1063 w1072]
          tunnel: [w1063 w1073] -> w982
          tunnel: [w1064 w1072] -> w981
          tunnel: w958 -> [w1062 w1070]
          tunnel: [w1062 w1068] -> _
          tunnel: w975 -> [_ w1071]
          frame False {
          }
          frame True {
            n395 = local read "No of Series"() -> (w1067:i32)
            n396 = Add(x=0.65, y=w1067) -> (x+y=w1066:dbl)
            n397 = Multiply(x=w1071, y=w1066) -> (x*y=w1069:dbl)
            n398 = Subtract(x=w1070, y=w1069) -> (x-y=w1068:dbl)
          }
        }
        n399 = call "Number_2_string.vi"("number"=w957) -> ("String"=w956:string)  [unwired: 1 in]
        n400 = case shown="True" w959 {
          tunnel: w958 -> [w997 w999]
          tunnel: [w997 w998] -> w954
          frame False {
          }
          frame True {
            n401 = Power Of 10(x=w999) -> (10^x=w998:dbl)
          }
        }
        n402 = call "Number_2_string.vi"("number"=w954) -> ("String"=w955:string)  [unwired: 1 in]
        n403 = Format Into String(format string="\n%sset key %s, %s\n%s unset key\n", initial string=w992, w982, w956, w955, w981) -> (resulting string=w993:string)  [unwired: 1 in, 1 out]
      }
      frame "Add Labels to plot" {
        n404 = stacked-sequence {
          seq-local: [w1083 _] -> [_ w1117]
          tunnel: [_ w1118] -> w1080
          tunnel: w1079 -> [_ w1119]
          tunnel: [_ "Set plot ranges" ("t")] -> w1076
          tunnel: w1075 -> [w1086 _]
          tunnel: w1074 -> [_ w1114]
          frame #0 {
            n405 = local read "Added labels"() -> (w1088:i32[])
            n406 = Index Array(array=w1086, index (col)=0 ("disabled index (col)")) -> (element=w1087:string[])  [unwired: 1 in]
            n407 = for {
              tunnel: w1088 -> [w1103] mode=indexing
              tunnel: w1087 -> [w1108]
              tunnel: w1086 -> [w1107]
              tunnel: "Summarise" -> [w1106]
              shift-right: [w1091] -> w1083
              shift-left: string[] [] -> [w1092]
              n408 = Add(x=w1106, y=u16 2) -> (x+y=w1104:u16)
              n409 = Index Array(array=w1107, index (col)=w1104) -> (element=w1102:string[])  [unwired: 1 in]
              n410 = Index Array(array=w1108, index=w1103) -> (element=w1098:string)
              n411 = Index Array(array=w1102, index=w1103) -> (element=w1095:string)
              n412 = call "Fast_string_Replace.vi"("Replace match with:"=" ", "Input String"=w1098, "regular expression"=":") -> ("Output String"=w1097:string)  [unwired: 1 in, 1 out]
              n413 = call <vilib>:"Trim Whitespace.vi"("string"=w1097) -> ("trimmed string"=w1096:string)  [unwired: 1 in]
              n414 = Format Into String(format string="%s = %s", w1096, w1095) -> (resulting string=w1090:string)  [unwired: 2 in, 1 out]
              n415 = Match Pattern(string=w1095, regular expression=";") -> (offset past match=w1093:i32)  [unwired: 1 in, 3 out]
              n416 = case shown="-1" w1093 {
                tunnel: w1092 -> [w1109 w1112]
                tunnel: [w1109 w1110] -> w1091
                tunnel: w1090 -> [_ w1111]
                frame 0, Default {
                }
                frame -1 {
                  n417 = Build Array (concatenate)(w1112, w1111) -> (w1110:string[])
                }
              }
            }
          }
          frame #1 {
            n418 = local read "Show legend?"() -> (w1113:bool)
            n419 = local read "X location"() -> (w1116:dbl)
            n420 = local read "Delta y"() -> (w1115:dbl)
            n421 = for {
              shift-right: [w1140] -> w1118
              shift-left: w1119 -> [w1141]
              tunnel: w1117 -> [w1137] mode=indexing
              tunnel: w1116 -> [w1129]
              tunnel: w1115 -> [w1142]
              tunnel: w1114 -> [w1136]
              tunnel: w1113 -> [w1122]
              i -> [w1143]
              n422 = call "Text_for_latex.vi"("Input String"=w1137) -> ("Output String"=w1131:string)
              n423 = String Length(string=w1131) -> (length=w1134:i32)
              n424 = Less?(x=w1134, y=20) -> (x < y?=w1123:bool)
              n425 = Compound Arithmetic op=AND(w1123, invert w1122) -> (w1121:bool)
              n426 = Increment(x=w1143) -> (x+1=w1144:i32)
              n427 = case shown="True" w1121 {
                tunnel: [w1146 w1148] -> w1132
                tunnel: w1131 -> [w1146 w1149]
                tunnel: "~~~~~~~~~~~" -> [_ w1147]
                frame False {
                }
                frame True {
                  n428 = Concatenate Strings(w1147, w1149) -> (w1148:string)
                }
              }
              n429 = Multiply(x=w1143, y=w1142) -> (x*y=w1138:dbl)
              n430 = local read "Y location"() -> (w1139:dbl)
              n431 = call "Number_2_string.vi"("precision"="2", "number"=w1129) -> ("String"=w1128:string)
              n432 = Subtract(x=w1139, y=w1138) -> (x-y=w1135:dbl)
              n433 = case shown="False" w1136 {
                tunnel: w1135 -> [w1150 w1152]
                tunnel: [w1150 w1151] -> w1127
                frame False {
                }
                frame True {
                  n434 = Power Of 10(x=w1152) -> (10^x=w1151:dbl)
                }
              }
              n435 = call "Number_2_string.vi"("precision"="2", "number"=w1127) -> ("String"=w1126:string)
              n436 = Format Into String(format string="set label %d '%s' at %s, %s\n", initial string=w1141, w1144, w1132, w1128, w1126) -> (resulting string=w1140:string)  [unwired: 1 in, 1 out]
            }
          }
        }
      }
      frame "Set plot ranges" {
        (unwired) "set border"
        (unwired) "set nologscale  y"
        (unwired) "set logscale  y"
        w1159 = ""
        n437 = property on="XY Graph" class="XYGraph (strict)"() -> ("X Scale.Range:Maximum"=w1177:dbl, "X Scale.Range:Minimum"=w1176:dbl, "Y Scale.Range:Maximum"=w1163:dbl, "Y Scale.Range:Minimum"=w1172:dbl)  [unwired: 2 in, 2 out]
        n438 = local read "Extra range"() -> (w1170:dbl)
        n439 = local read "Profile offset"() -> (w1166:dbl)
        n440 = Select(t="\nset logscale  y\n", s=w1161, f=w1159) -> (s? t:f=w1157:string)
        n441 = Decrement(x=w1165) -> (x-1=w1167:dbl)
        n442 = case shown="False" w1182 {
          tunnel: w1159 -> [w1194 w1196]
          tunnel: [w1194 w1195] -> w1184
          tunnel: "#" -> [w1193 w1195]
          tunnel: [w1193 w1196] -> w1183
          frame False {
          }
          frame True {
          }
        }
        n443 = Multiply(x=w1166, y=w1167) -> (x*y=w1164:dbl)
        n444 = Add(x=w1164, y=w1163) -> (x+y=w1162:dbl)
        n445 = Subtract(x=w1172, y=w1170) -> (x-y=w1171:dbl)
        n446 = call "Number_2_string.vi"("number"=w1162) -> ("String"=w1155:string)  [unwired: 1 in]
        n447 = call "Number_2_string.vi"("number"=w1171) -> ("String"=w1156:string)  [unwired: 1 in]
        n448 = case shown="\"Linespoints\"" w1180 {
          tunnel: ["Plot Command" "Plot Command" "Plot Command" "Calculate fit parameters"] -> w1179
          frame "None" {
          }
          frame "Linespoints" {
          }
          frame "Spline" {
          }
          frame "Linear", Default {
          }
        }
        n449 = call "Number_2_string.vi"("number"=w1177) -> ("String"=w1153:string)  [unwired: 1 in]
        n450 = call "Gnuplot_offset_ytics.vi"("Separation"=w1165, "Mode"="Mode", "precision"="precision", "Legend"=w1168, "Max Plot Value"=w1163, "Profile offset"=w1166) -> ("concatenated string"=w1158:string)
        n451 = call "Number_2_string.vi"("number"=w1176) -> ("String"=w1154:string)  [unwired: 1 in]
        n452 = Format Into String(format string="%s set xrange [%s : %s] \n%s set autoscale x \n%s set yrange [%s : %s]\n%s set autoscale y \n", initial string=w1181, w1184, w1154, w1153, w1183, w1184, w1156, w1155, w1183) -> (resulting string=w1174:string)  [unwired: 1 in, 1 out]
        n453 = Concatenate Strings(w1174, w1157, w1158) -> (w1175:string)
      }
      frame "Calculate fit parameters" {
        # "k=1;    # label 1\nlab=\"23 mA\";\neval( sprintf (\"set label %d %s\", k, lab))"
        n454 = Strip Path(path=w1202) -> (name=w1201:string)  [unwired: 1 out]
        n455 = for {
          tunnel: w1204 -> [w1211]
          tunnel: w1201 -> [w1209]
          shift-right: [w1207] -> w1199
          shift-left: w1200 -> [w1208]
          tunnel: w1197 -> [w1206] mode=indexing
          i -> [w1210]
          n456 = case shown="\"Gaussian\"" w1211 {
            tunnel: w1210 -> [w1213 w1228 w1231 w1236 w1241 _]
            tunnel: w1209 -> [w1212 w1229 w1232 w1237 w1242 _]
            tunnel: w1208 -> [w1224 w1227 w1234 w1239 w1244 w1246]
            tunnel: [w1223 w1226 w1233 w1238 w1243 w1246] -> w1207
            tunnel: w1206 -> [w1222 _ _ _ _ _]
            frame "Gaussian" {
              n457 = Unbundle(w1222) -> ("Output"=w1220:dbl[], "Pwr out"=w1221:dbl[])
              n458 = Array Max & Min(array=w1221) -> (max value=w1215:dbl)  [unwired: 3 out]
              n459 = Array Max & Min(array=w1220) -> (max value=w1219:dbl, min value=w1218:dbl)  [unwired: 2 out]
              n460 = Subtract(x=w1219, y=w1218) -> (x-y=w1217:dbl)
              n461 = Divide(x=w1217, y=6.0) -> (x/y=w1214:dbl)
              n462 = Format Into String(format string="\nf%d(x) = cmax%d*exp(-((x-offset%d)**2)/(2*sig%d**2))\ncmax%d = %.2f; sig%d = %.2f; offset%d = 1           # initial guess for cmax and sig and offset\nfit f%d(x) \"%s.dat\" index %d using 1:2 via cmax%d, sig%d, offset%d #this is a gaussian fit\n", initial string=w1224, w1213, w1213, w1213, w1213, w1213, w1215, w1213, w1214, w1213, w1213, w1212, w1213, w1213, w1213, w1213) -> (resulting string=w1223:string)  [unwired: 1 in, 1 out]
            }
            frame "2nd Ploy" {
              n463 = Format Into String(format string="\nf%d(x) = c%d*x**2 + b%d*x + a%d\n#a%d = 40; b%d = 300; c%d = 1           # initial guess for cmax and sig and offset\nfit f%d(x) \"%s.dat\" index %d using 1:2 via a%d, b%d, c%d #this is a 2nd order poly fit\n", initial string=w1227, w1228, w1228, w1228, w1228, w1228, w1228, w1228, w1228, w1229, w1228, w1228, w1228, w1228) -> (resulting string=w1226:string)  [unwired: 1 in, 1 out]
            }
            frame "3rd Poly" {
              n464 = Format Into String(format string="\nf%d(x) = d%d*x**3 +c%d*x**2 + b%d*x + a%d\n#a%d = 40; b%d = 300; c%d = 1; d%d = 1         # initial guess for cmax and sig and offset\nfit f%d(x) \"%s.dat\" index %d using 1:2 via a%d, b%d, c%d, d%d #this is a 3rd order poly fit\n", initial string=w1234, w1231, w1231, w1231, w1231, w1231, w1231, w1231, w1231, w1231, w1231, w1232, w1231, w1231, w1231, w1231, w1231) -> (resulting string=w1233:string)  [unwired: 1 in, 1 out]
            }
            frame "4th Poly" {
              n465 = Format Into String(format string="\nf%d(x) = e%d*x**4 + d%d*x**3 +c%d*x**2 + b%d*x + a%d\n#a%d = 40; b%d = 300; c%d = 1; d%d = 1  e%d = 1       # initial guess for cmax and sig and offset\nfit f%d(x) \"%s.dat\" index %d using 1:2 via a%d, b%d, c%d, d%d, e%d #this is a 3rd order poly fit\n", initial string=w1239, w1236, w1236, w1236, w1236, w1236, w1236, w1236, w1236, w1236, w1236, w1236, w1236, w1237, w1236, w1236, w1236, w1236, w1236, w1236) -> (resulting string=w1238:string)  [unwired: 1 in, 1 out]
            }
            frame "Linear" {
              n466 = Format Into String(format string="\nf%d(x) = b%d*x + c%d\n#a%d = 40; b%d = 300; c%d = 1           # initial guess for cmax and sig and offset\nfit f%d(x) \"%s.dat\" index %d using 1:2 via b%d, c%d #this is a Linear fit\n", initial string=w1244, w1241, w1241, w1241, w1241, w1241, w1241, w1241, w1242, w1241, w1241, w1241) -> (resulting string=w1243:string)  [unwired: 1 in, 1 out]
            }
            frame "Spline", Default {
            }
          }
        }
      }
      frame "Plot Command" {
        n467 = local read "No of Series"() -> (w1265:i32)
        n468 = Strip Path(path=w1262) -> (name=w1264:string)  [unwired: 1 out]
        n469 = for {
          N: w1265 -> [_]
          shift-right: [w1285] -> w1254
          shift-left: "\nplot " -> [w1286]
          tunnel: w1264 -> [w1287]
          tunnel: w1251 -> [w1284]
          tunnel: w1261 -> [w1270] mode=indexing
          tunnel: "Plot style" -> [w1277]
          shift-right: [w1272] -> _
          shift-left: 0 -> [w1274]
          tunnel: w1249 -> [w1269]
          shift-right: [w1267] -> _
          shift-left: 1 -> [w1268]
          i -> [w1276]
          n470 = Index Array(array=w1277, index=w1276) -> (element=w1275:u16)
          n471 = case shown="1" w1275 {
            tunnel: w1274 -> [w1290 w1298 w1305]
            tunnel: [w1297 w1298 w1305] -> w1272
            tunnel: [w1294 w1301 "linespoints, "] -> w1271
            tunnel: w1269 -> [w1296 _ _]
            tunnel: w1268 -> [w1289 w1299 w1303]
            tunnel: [w1289 w1300 w1303] -> w1267
            frame 0, Default {
              n472 = Increment(x=w1290) -> (x+1=w1297:i32)
              n473 = Quotient & Remainder(x=w1290, y=8) -> (x-y*floor(x/y)=w1292:i32)  [unwired: 1 out]
              n474 = Index Array(array=w1296, index=w1292) -> (element=w1295:i32)
              n475 = Format Into String(format string="points 1 %d, ", w1295) -> (resulting string=w1294:string)  [unwired: 2 in, 1 out]
            }
            frame 1 {
              n476 = Increment(x=w1299) -> (x+1=w1300:i32)
              n477 = Format Into String(format string="lines lt %d, ", w1299) -> (resulting string=w1301:string)  [unwired: 2 in, 1 out]
            }
            frame 2 {
            }
          }
          n478 = case shown="\"Spline\"" w1284 {
            tunnel: w1276 -> [_ w1313 w1317 w1320 w1323 w1326 w1329]
            tunnel: w1287 -> [_ w1315 _ _ _ _ _]
            tunnel: ["" w1314 w1318 w1321 w1324 w1327 w1330] -> w1283
            frame "None", Default {
            }
            frame "Spline" {
              n479 = Quotient & Remainder(x=w1313, y=2) -> (x-y*floor(x/y)=w1311:i32)  [unwired: 1 out]
              n480 = Equal To 0?(x=w1311) -> (x = 0?=w1310:bool)
              n481 = Select(t="1", s=w1310, f="2") -> (s? t:f=w1307:string)
              n482 = Format Into String(format string="\"%s.dat\" index %d using 1:2 axes x1y1 title '' lt %s smooth csplines, ", w1315, w1313, w1307) -> (resulting string=w1314:string)  [unwired: 2 in, 1 out]
            }
            frame "Gaussian" {
              n483 = Format Into String(format string="cmax%d*exp(-((x-offset%d)**2)/(2*sig%d**2)) title 'fit%d', ", w1317, w1317, w1317, w1317) -> (resulting string=w1318:string)  [unwired: 2 in, 1 out]
            }
            frame "2nd Ploy" {
              n484 = Format Into String(format string="c%d*x**2 + b%d*x + a%d title 'fit%d', ", w1320, w1320, w1320, w1320) -> (resulting string=w1321:string)  [unwired: 2 in, 1 out]
            }
            frame "3rd Poly" {
              n485 = Format Into String(format string="d%d*x**3  + c%d*x**2 + b%d*x + a%d title 'fit%d', ", w1323, w1323, w1323, w1323, w1323) -> (resulting string=w1324:string)  [unwired: 2 in, 1 out]
            }
            frame "4th Poly" {
              n486 = Format Into String(format string="e%d*x**4 + d%d*x**3  + c%d*x**2 + b%d*x + a%d title 'fit%d', ", w1326, w1326, w1326, w1326, w1326, w1326) -> (resulting string=w1327:string)  [unwired: 2 in, 1 out]
            }
            frame "Linear" {
              n487 = Format Into String(format string="b%d*x + c%d title 'fit%d', ", w1329, w1329, w1329) -> (resulting string=w1330:string)  [unwired: 2 in, 1 out]
            }
          }
          n488 = call "Fast_string_Replace.vi"("Replace match with:"="", "Input String"=w1270, "regular expression"="[$]") -> ("Output String"=w1278:string)  [unwired: 1 in, 1 out]
          n489 = Format Into String(format string="\"%s.dat\" index %d using 1:2 axes x1y1 title '$%s$' with ", initial string=w1286, w1287, w1276, w1278) -> (resulting string=w1273:string)  [unwired: 1 in, 1 out]
          n490 = Concatenate Strings(w1273, w1271, w1283, "\\" ("string"), "\n") -> (w1285:string)
        }
        n491 = String Length(string=w1254) -> (length=w1258:i32)
        n492 = Subtract(x=w1258, y=4) -> (x-y=w1256:i32)
        n493 = String Subset(string=w1254, length (rest)=w1256) -> (substring=w1255:string)  [unwired: 1 in]
        n494 = Concatenate Strings(w1260, w1255) -> (w1259:string)
      }
      frame "Write gnuplot file" {
        w1339 = "\n"
        w1343 = FALSE  # append to file? (new file:F)
        w1344 = FALSE  # advisory dialog? (display:T)
        n495 = Strip Path(path=w1335) -> (stripped path=w1346:path)  [unwired: 1 out]
        n496 = Build Path(base path=w1346, name or relative path="gnuplot_script.txt") -> (appended path=w1345:path)
        n497 = call "gnuplot_legend.vi"("Plot style"=w1332, "Legend"=w1336) -> ("Tex String"=w1340:string)
        n498 = Concatenate Strings(w1337, w1339, w1339, "#" ("string"), w1340) -> (w1342:string)
        n499 = call "Write_Characters_To_File.vi"("file path (dialog if empty)"=w1345, "advisory dialog? (display:T)"=w1344, "character string"=w1342, "append to file? (new file:F)"=w1343) -> ()  [unwired: 4 in, 1 out]
      }
      frame "Execute shell script" {
        w1350 = FALSE  # append to file? (new file:F)
        w1351 = FALSE  # advisory dialog? (display:T)
        w1361 = TRUE  # wait until completion? (T)
        n500 = Strip Path(path=w1354) -> (stripped path=w1349:path, name=w1360:string)
        n501 = Build Path(base path=w1349, name or relative path=w1348) -> (appended path=w1353:path)
        n502 = Format Into String(format string="/usr/local/bin/data2eps.sh \"%s\"", w1360) -> (resulting string=w1358:string)  [unwired: 2 in, 1 out]
        n503 = call <vilib>:"System Exec.vi"("wait until completion? (T)"=w1361, "working directory"=w1349, "command line"=w1358) -> ("standard output"=w1352:string)  [unwired: 5 in, 3 out]
        n504 = call "Write_Characters_To_File.vi"("file path (dialog if empty)"=w1353, "character string"=w1352, "append to file? (new file:F)"=w1350, "Lock File"=w1351) -> ()  [unwired: 4 in, 1 out]
      }
      frame "Has pdf been generated?" {
        n505 = Strip Path(path=w1368) -> (stripped path=w1370:path, name=w1372:string)
        n506 = Concatenate Strings(w1372, ".pdf" ("string")) -> (w1371:string)
        n507 = Build Path(base path=w1370, name or relative path=w1371) -> (appended path=w1367:path)
        n508 = call "Does_file_exist_(simple).vi"("Pathname"=w1367) -> ("exists?"=w1365:bool)
        n509 = case shown="True" w1365 {
          tunnel: ["Open Standard output file" ("f") "Keep Plot?" ("t")] -> w1366
          frame False {
          }
          frame True {
          }
        }
      }
      frame "Keep Plot?" {
        n510 = Strip Path(path=w1387) -> (stripped path=w1379:path, name=w1391:string)
        n511 = Strip Path(path=w1379) -> (stripped path=w1382:path, name=w1381:string)
        n512 = Concatenate Strings(w1391, ".pdf" ("string")) -> (w1390:string)
        n513 = Build Path(base path=w1379, name or relative path=w1390) -> (appended path=w1388:path)
        n514 = Format Into String(format string="Do you want to keep\n%s", w1388) -> (resulting string=w1384:string)  [unwired: 2 in, 1 out]
        n515 = Two Button Dialog(message=w1384, 1:"Delete" ("F button name (\"Cancel\")"), 2:"Keep" ("T button name (\"OK\")")) -> (T button?=w1383:bool)
        n516 = case shown="False" w1383 {
          tunnel: w1382 -> [w1400 _]
          tunnel: w1381 -> [w1399 _]
          tunnel: w1378 -> [_ _]
          frame False {
            n517 = Format Into String(format string="rm -r %s", w1399) -> (resulting string=w1397:string)  [unwired: 2 in, 1 out]
            n518 = call <vilib>:"System Exec.vi"("working directory"=w1400, "command line"=w1397) -> ()  [unwired: 6 in, 4 out]
          }
          frame True {
          }
        }
      }
      frame "Open Standard output file" {
        n519 = Strip Path(path=w1405) -> (stripped path=w1402:path)  [unwired: 1 out]
        n520 = Format Into String(format string="open \"%s\"", w1403) -> (resulting string=w1401:string)  [unwired: 2 in, 1 out]
        n521 = call <vilib>:"System Exec.vi"("working directory"=w1402, "command line"=w1401) -> ()  [unwired: 6 in, 4 out]
      }
    }
  }
  "Tex Info String" <- w13
  "Saved Automatically?" <- FALSE
